vi "运维调试_总磷.vi"() -> ()   [LabVIEW 2016, in "斯坦道总磷.lvlib"]
uses:
  <vilib>/Utility/miscctls.llb/LVPointTypeDef.ctl
  <vilib>/Utility/config.llb/NI_LVConfig.lvlib
  <vilib>/ptbypt/NI_PtbyPt.lvlib
panel:
  in  "定时设置":cluster{"启动":bool, "控制命令":T1, "测量参数":T2}(xcontrol)
  in  "仪器参数设置":bool
  in  "模块启用":bool
  in  "串口设置":bool
  in  "备用系数一键写入":bool
  in  "公式一键写入":bool
  in  "流程路径":path=path "C:/Users/STD/Documents/斯坦道流程文件/流程.xml"
  in  "曲线模型":cluster{"X^2":dbl, "X":dbl, "B":dbl, "r^2":dbl}(xcontrol)
  out "字符串":string
  in  "质控参数设置":bool
  in  "总磷自动测试量程配置":T3
  out "温度2":sgl
  out "温度1":sgl
  out "ADC":sgl
  out "固件版本号":string
  in  "数组":string[](array[string])
  in  "备用系数写入":bool
  in  "备用系数读取":bool
  in  "备用系数":T4
  in  "量程切换阈值写入":bool
  in  "量程切换阈值读取":bool
  in  "量程切换阈值":cluster{"阈值":dbl, "标液浓度":dbl}
  in  "参数下拉列表":enum16{"总磷", "总氮"}(ring)
  in  "量程下拉列表":enum16{"低量程", "高量程"}(ring)
  in  "测量模式下拉列表":enum16{"水样测量", "零点核查", "跨度核查", "标样核查", "加标回收"}(ring)
  in  "公式":cluster{"X^2":dbl, "X":dbl, "b":dbl}
  in  "写公式":bool
  in  "读公式":bool
  in  "返回":bool
  in  "设置":bool
  out "序列号":string="序列号"
  out "测量数据":T5(xcontrol)
  out "集成报警信息":string
  out "总磷总氮运行状态":T6(xcontrol)
  in  "停止":bool
  in  "手动启动":bool
  in  "单步测试":bool
  in  "总磷氨氮调试":u16[](xcontrol)
  out "F3":sgl format="%#.6f"
  out "F2":sgl format="%#.6f"
  out "F1":sgl format="%#.6f"
  out "F0":sgl format="%#.6f"
  out "多列列表框":i32(listbox)
  # "参数设置"
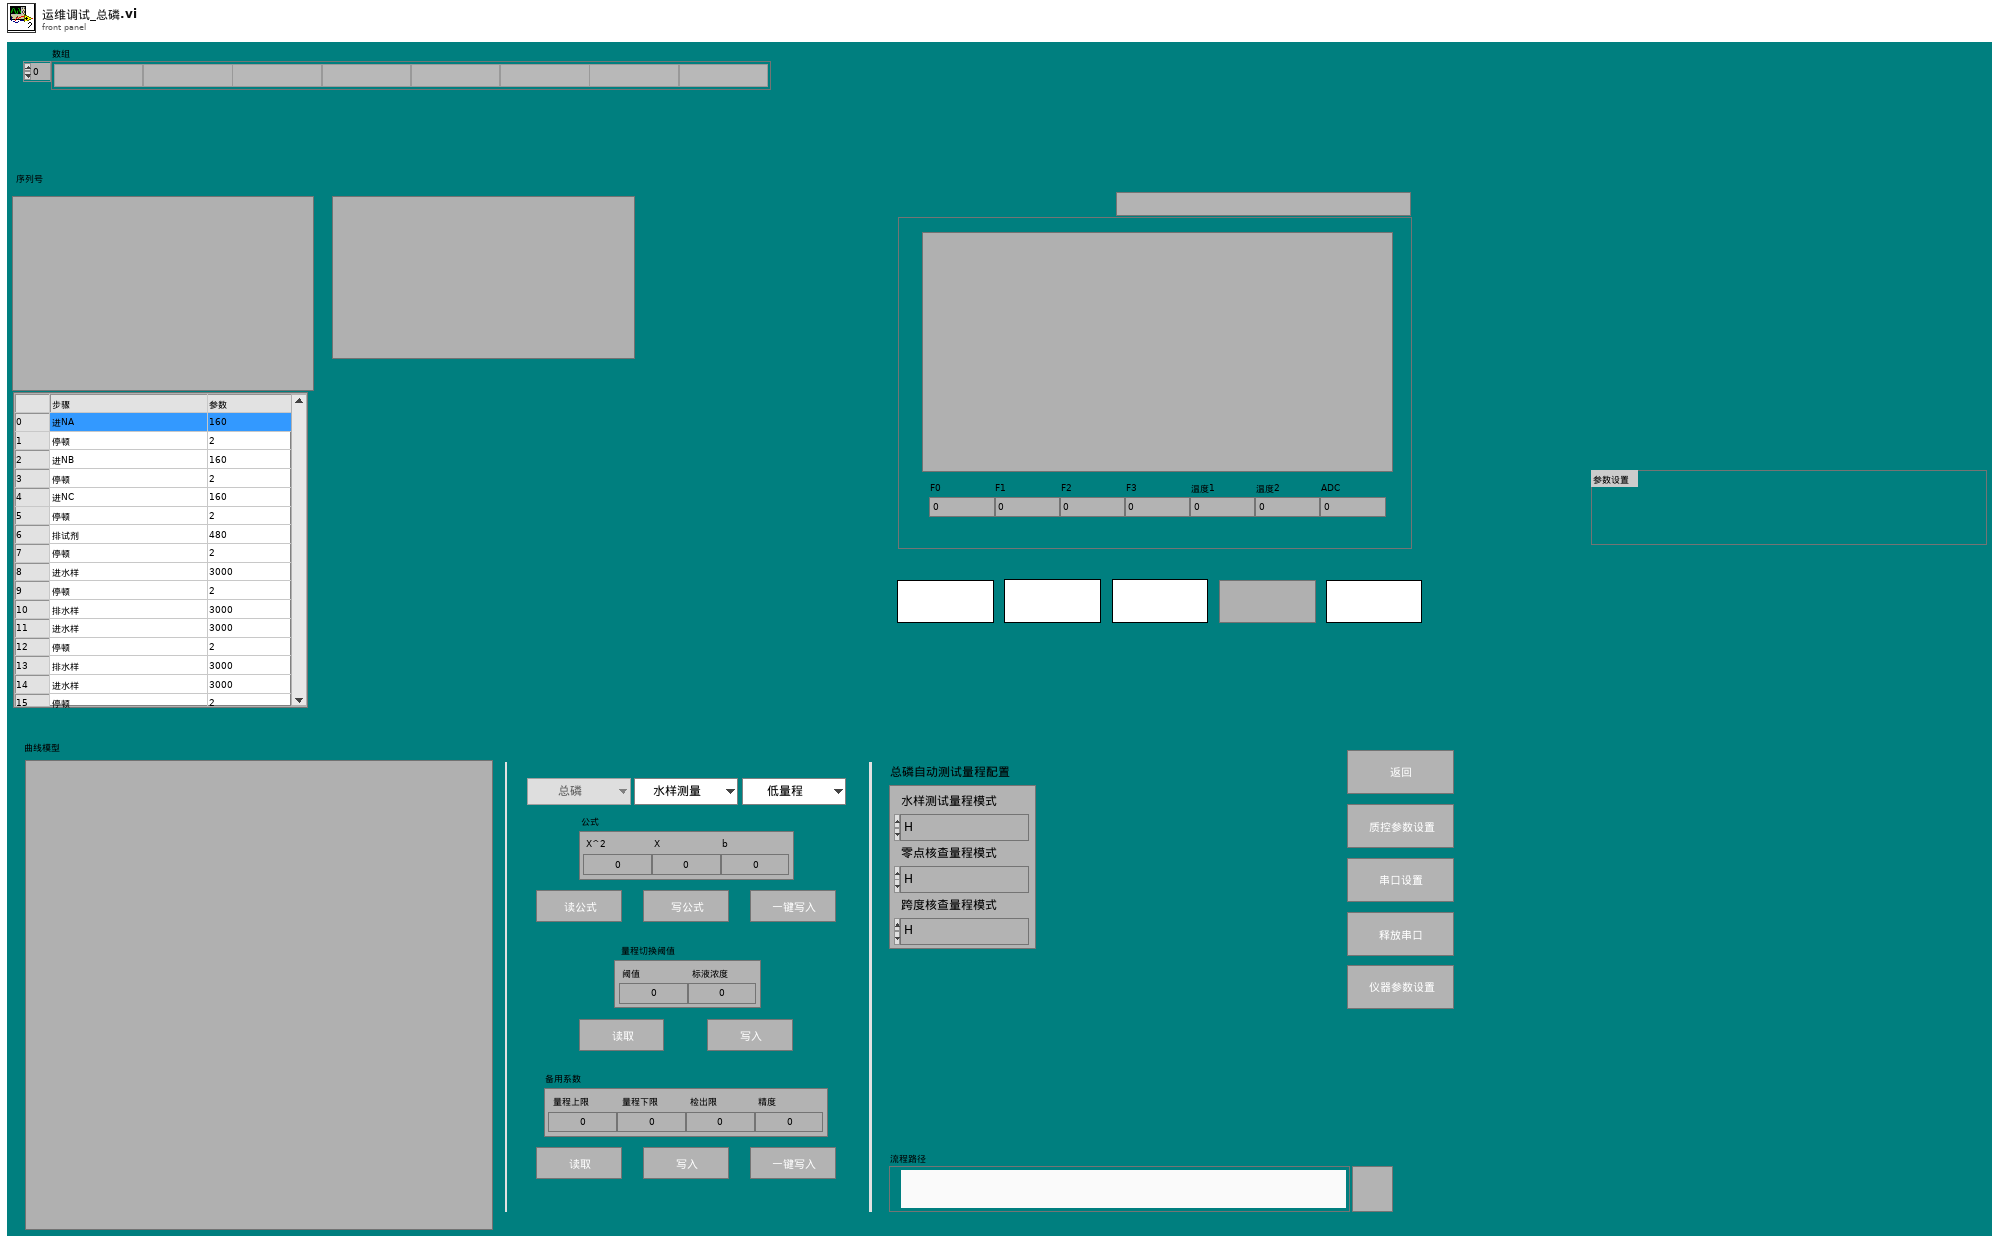
[diagram p1: front panel]
types:
  T1 = typedef "定时设置.xctl/国标控制命令.ctl" = enum16{"启动测量", "标样核查", "零点核查", "跨度核查", "空白测试", "平行样测试", "加标回收", "空白校准", "标样校准", "初始化（清洗）", "停止测试", "仪器重启", "校时", "模式设置", "测量间隔设置"}
  T2 = typedef "定时设置.xctl/测量参数.ctl" = u16
  T3 = cluster{"水样测试量程模式":enum16{"H", "L", "AUTO"}, "空白核查量程模式":enum16{"H", "L", "AUTO"}, "跨度核查量程模式":enum16{"H", "L", "AUTO"}}
  T4 = cluster{"量程上限":dbl, "量程下限":dbl, "检出限":dbl, "精度":dbl}
  T5 = cluster{"flowid":u16, "测量精度":u16, "测量数据区":cluster{"因子编码":u32, "单位":u16, "标样参考值":sgl, "水样数据时间":timestamp, "水样实测值":sgl, "水样数据标识":string, "标样数据时间":timestamp, "标样实测值":sgl, "标样数据标识":string, "空白数据时间":timestamp, "空白实测值":sgl, "空白数据标识":string, "零点核查数据时间":timestamp, "零点核查实测值":sgl, "零点核查数据标识":string, "跨度核查数据时间":timestamp, "跨度核查实测值":sgl, "跨度核查数据标识":string, "加标回收数据时间":timestamp, "加标回收实测值":sgl, "加标回收数据标识":string, "平行样数据时间":timestamp, "平行样实测值":sgl, "平行样数据标识":string, "F0":sgl, "F1":sgl, "F2":sgl, "F3":sgl, "F4":sgl, "F5":sgl, "F6":sgl, "F7":sgl, "温度":sgl, "湿度":sgl, "X值":sgl}}
  T6 = cluster{"系统时间":timestamp, "工作状态":enum16{"空闲", "水样测试", "标样核查", "零点核查", "跨度核查", "空白测试", "平行样测试", "加标回收", "空白校准", "标样校准", "初始化（清洗）"}, "测量模式":enum16{"待机", "连续模式", "周期模式", "定点模式", "受控模式", "手动模式"}, "告警代码":u16, "故障代码":u16, "日志代码":u16, "软件版本":u16, "F0":sgl, "F1":sgl, "F2":sgl, "F3":sgl, "T":sgl, "H":sgl, "id":u16, "flowid":u16, "量程":u16, "总磷控温温度1":sgl, "营养盐控温温度2":sgl, "ADC":sgl}
  T7 = typedef "NI_LVConfig.lvlib/Config Data RefNum.ctl" = refnum<k1>
  T8 = typedef "LVPointTypeDef.ctl" = cluster{"Horizontal":i16, "Vertical":i16}
  T9 = enum16{"空闲", "水样测试", "标样核查", "零点核查", "跨度核查", "空白测试", "平行样测试", "加标回收", "空白校准", "标样校准", "初始化（清洗）"}
  T10 = cluster{"因子编码":u32, "单位":u16, "标样参考值":sgl, "水样数据时间":timestamp, "水样实测值":sgl, "水样数据标识":string, "标样数据时间":timestamp, "标样实测值":sgl, "标样数据标识":string, "空白数据时间":timestamp, "空白实测值":sgl, "空白数据标识":string, "零点核查数据时间":timestamp, "零点核查实测值":sgl, "零点核查数据标识":string, "跨度核查数据时间":timestamp, "跨度核查实测值":sgl, "跨度核查数据标识":string, "加标回收数据时间":timestamp, "加标回收实测值":sgl, "加标回收数据标识":string, "平行样数据时间":timestamp, "平行样实测值":sgl, "平行样数据标识":string, "F0":sgl, "F1":sgl, "F2":sgl, "F3":sgl, "F4":sgl, "F5":sgl, "F6":sgl, "F7":sgl, "温度":sgl, "湿度":sgl, "X值":sgl}
  T11 = cluster{"时间源选择":enum16{"系统时间源", "仪器时间源"}, "外部时间源":timestamp}
  T12 = enum32{"Bad", "Idle", "Run top level", "Running"}
  T13 = cluster{"参数下拉列表":enum16{"总磷", "总氮"}, "测量模式下拉列表":enum16{"水样测量", "零点核查", "跨度核查", "标样核查", "加标回收"}, "量程下拉列表":enum16{"低量程", "高量程"}}
  T14 = cluster{"启动模式":enum16{"跨度核查", "水样测量", "空白核查", "标样核查", "加标回收"}, "启动参数":u16, "量程":enum16{"低量程", "高量程"}}
  T15 = cluster{"时间标识":timestamp, "设备":string, "日志信息":string, "流程参数":string}
  T16 = cluster{"时间标识":timestamp, "设备":string, "日志信息":string}
  T17 = typedef "LVRowAndColumnUnsignedTypeDef.ctl" = cluster{"Row":u32, "Column":u32}
  T18 = enum8{"Enabled", "Disabled", "Disabled and Grayed Out"}
  T19 = cluster{"站号":u16, "量程切换":enum32{"H", "L", "AUTO"}, "控制命令":enum16{"启动测量", "标样核查", "零点核查", "跨度核查", "空白测试", "平行样测试", "加标回收", "空白校准", "标样校准", "初始化（清洗）", "停止测试", "仪器重启", "校时", "模式设置", "测量间隔设置"}, "模式设置":enum16{"待机", "连续模式", "周期模式", "定点模式", "受控模式", "手动模式"}, "测量间隔":u16}
  T20 = cluster{"总磷跨度值":dbl, "总磷零点标准液浓度":dbl, "总磷跨度标准液浓度":dbl, "总磷标准液标准浓度":dbl}
  T21 = cluster{"确定":bool, "总磷跨度值":dbl, "总磷零点标准液浓度":dbl, "总磷跨度标准液浓度":dbl, "总磷标准液标准浓度":dbl}
  T22 = cluster{"测量量程":dbl, "测量精度":dbl, "测量间隔":dbl, "消解温度":dbl, "消解时长":dbl, "空白校准时间":timestamp, "曲线截距":dbl, "曲线斜率":dbl, "测量检出限":dbl, "测量信号值":dbl, "线性相关系数":dbl, "二次多项式系数":dbl, "标样校准时间":timestamp, "稀释倍数":dbl, "三项式系数":dbl, "空白标定系数":dbl, "量程系数":dbl, "F0/ORPA":dbl, "F1/ORPB":dbl, "F2/ORPK":dbl, "F3":dbl, "F4":dbl, "F5":dbl, "F6":dbl, "F7":dbl, "X0/滴定数":dbl, "量程":dbl}
  T23 = cluster{"确定":bool, "测量量程":dbl, "测量精度":dbl, "测量间隔":dbl, "消解温度":dbl, "消解时长":dbl, "空白校准时间":timestamp, "曲线截距":dbl, "曲线斜率":dbl, "测量检出限":dbl, "测量信号值":dbl, "线性相关系数":dbl, "二次多项式系数":dbl, "标样校准时间":timestamp, "稀释倍数":dbl, "三项式系数":dbl, "空白标定系数":dbl, "量程系数":dbl, "F0/ORPA":dbl, "F1/ORPB":dbl, "F2/ORPK":dbl, "F3":dbl, "F4":dbl, "F5":dbl, "F6":dbl, "F7":dbl, "X0/滴定数":dbl, "量程":dbl}
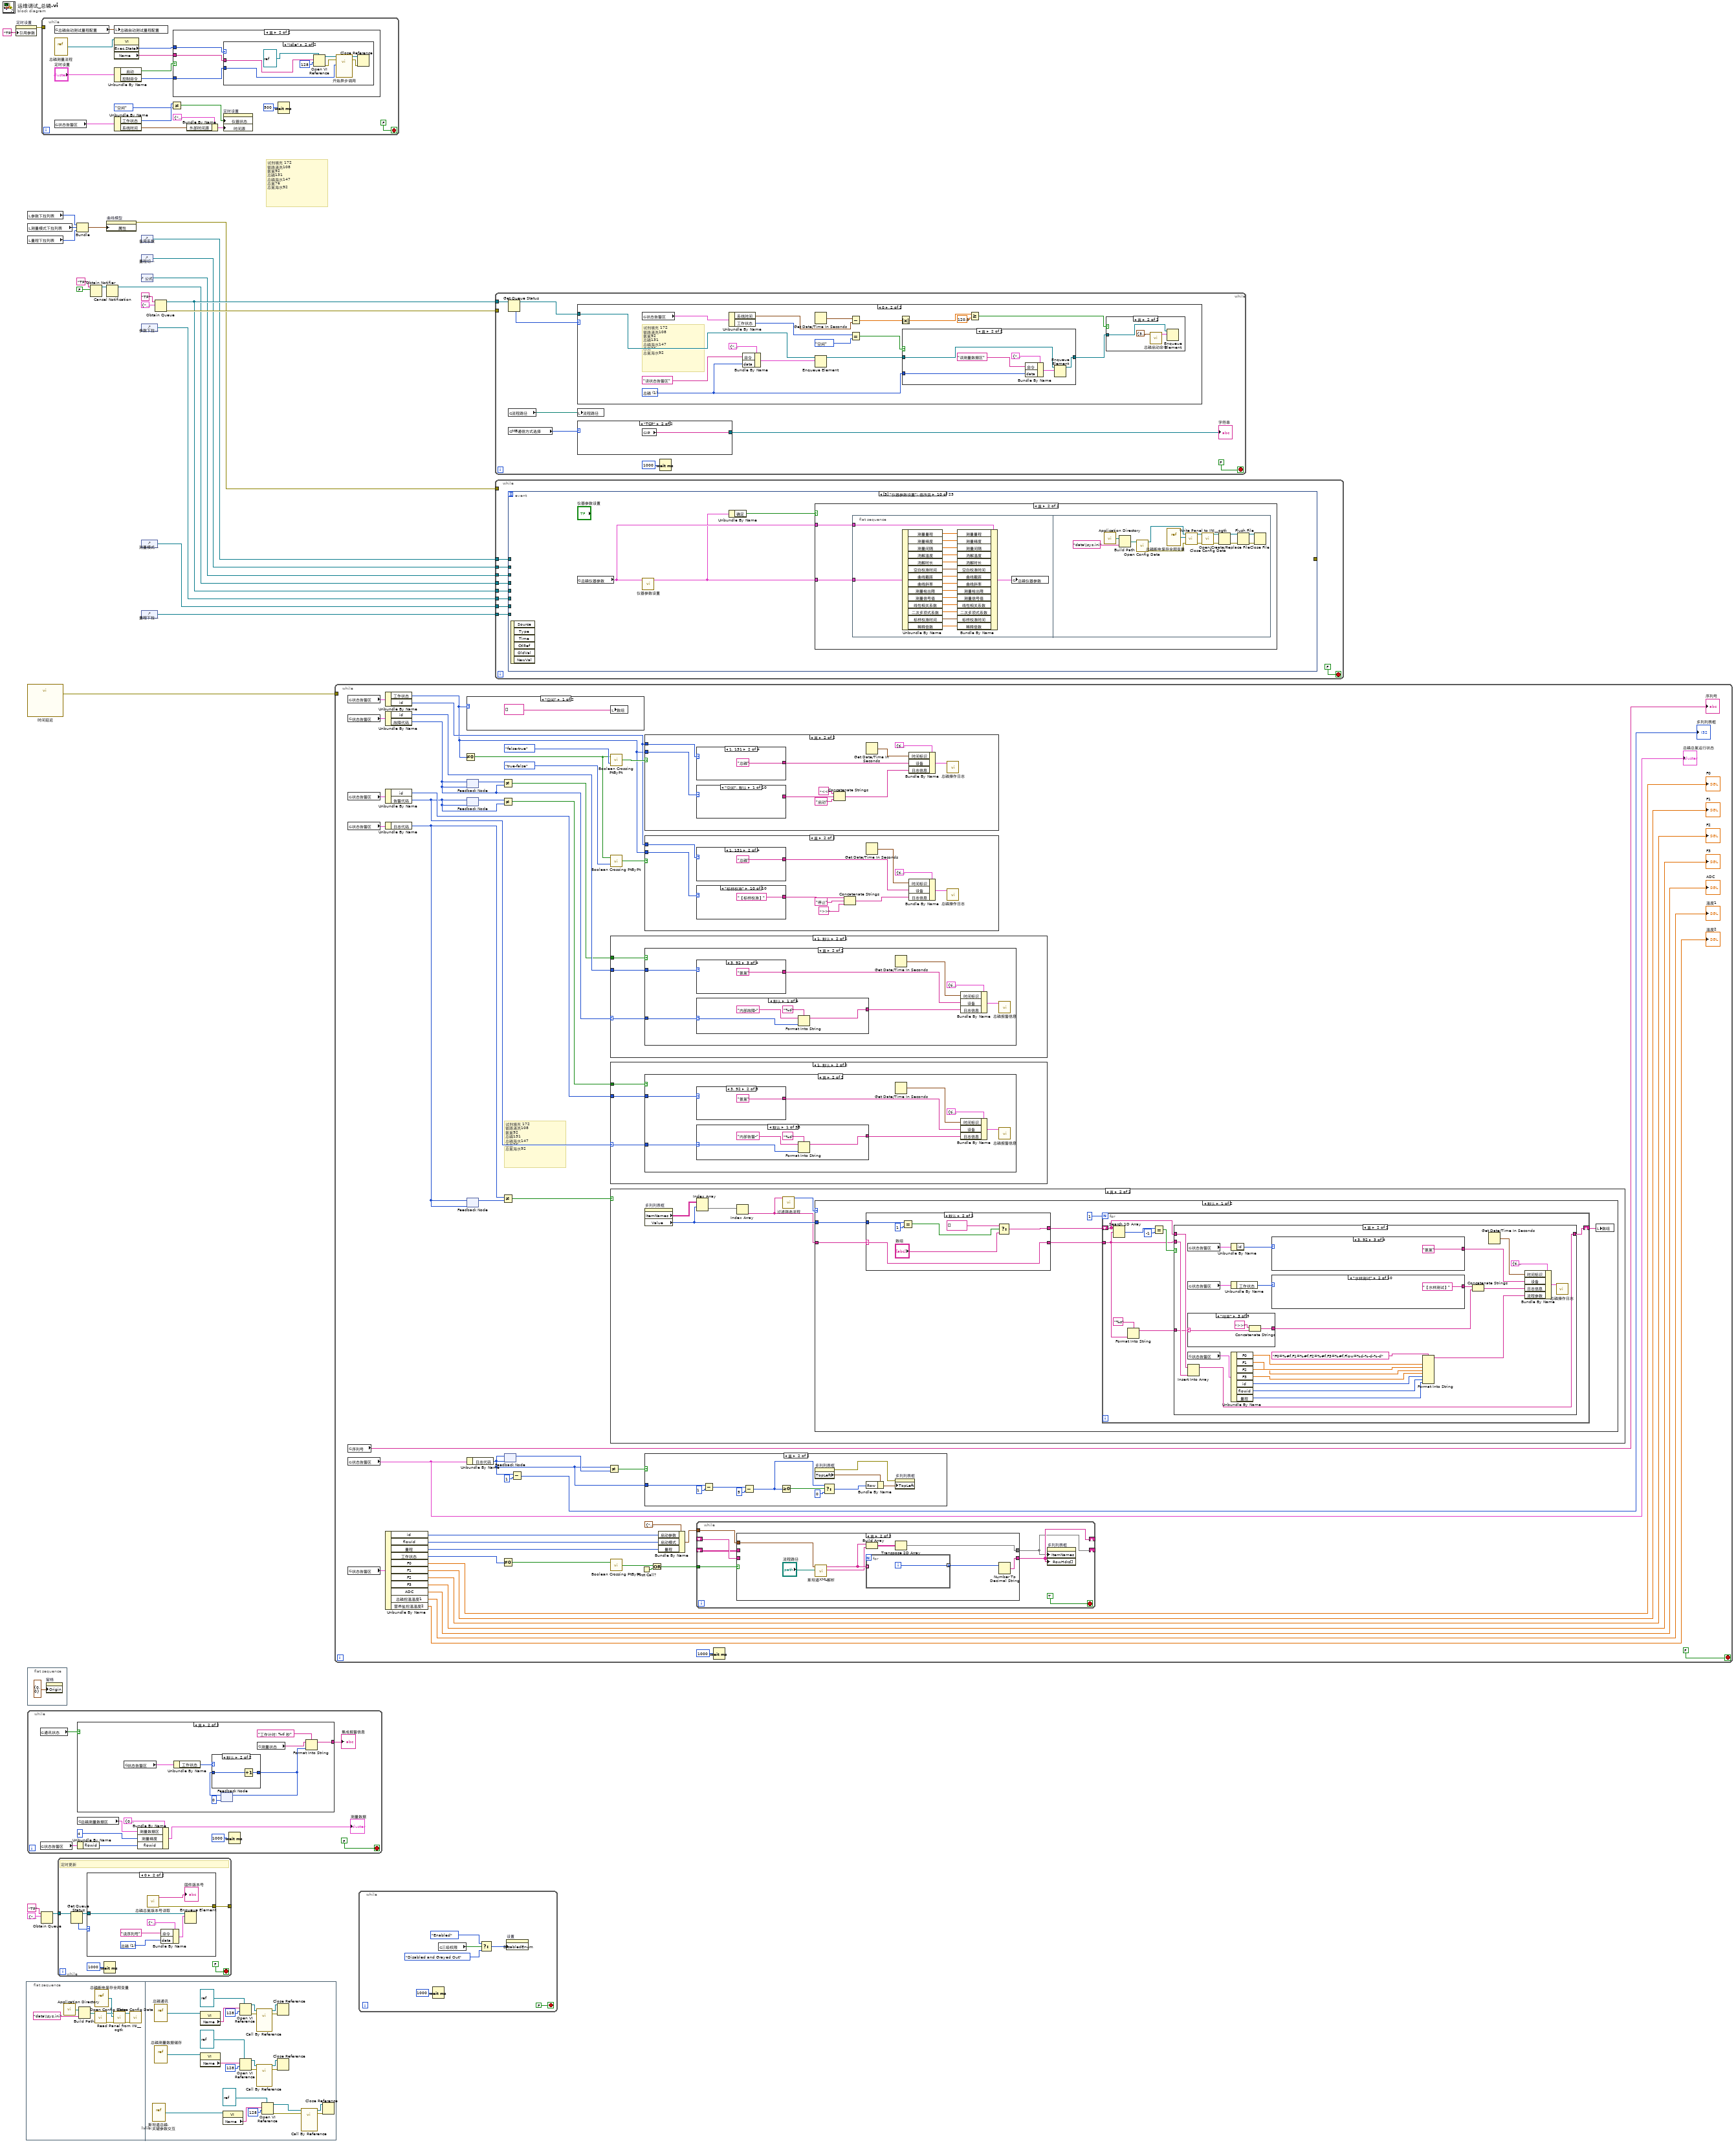
[diagram p0: block diagram]
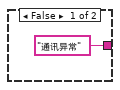
[diagram p3: hidden frame]
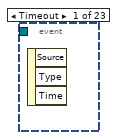
[diagram p7: hidden frame]
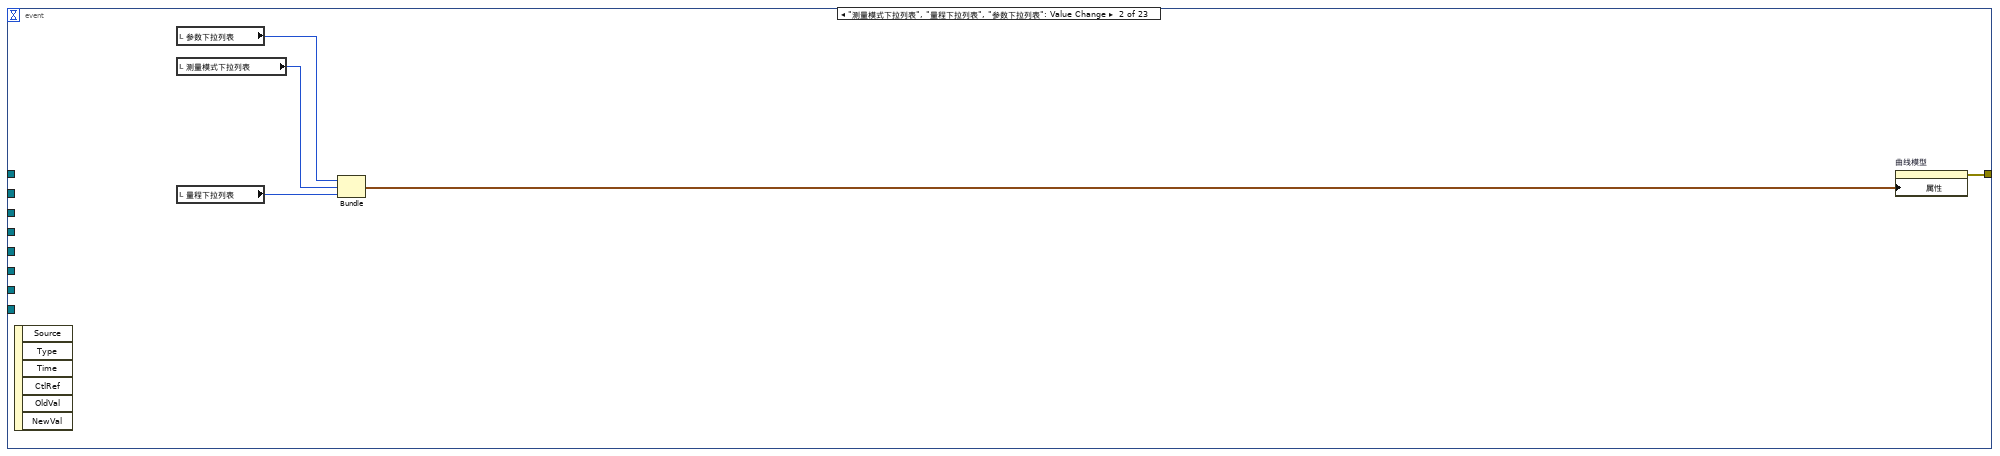
[diagram p8: hidden frame]
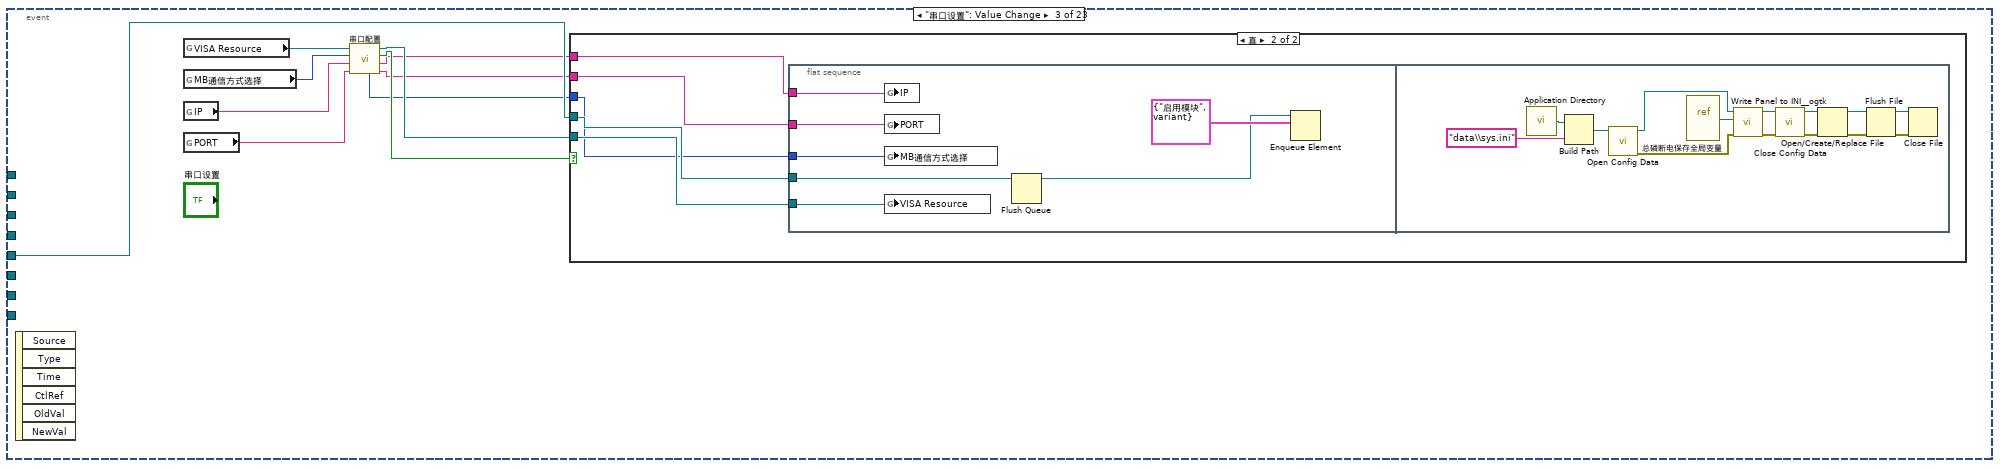
[diagram p9: hidden frame]
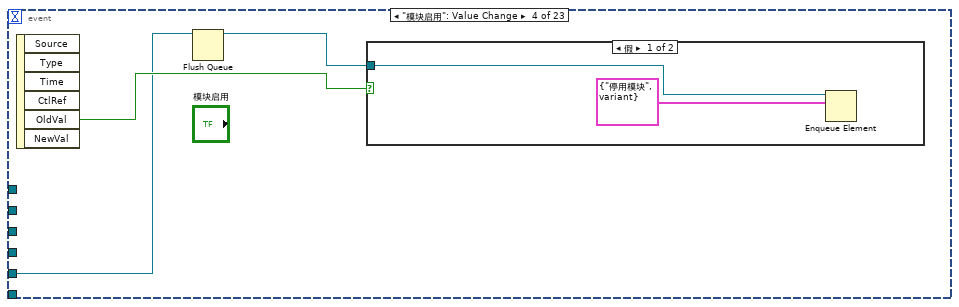
[diagram p11: hidden frame]
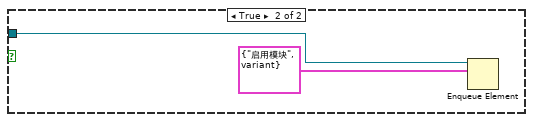
[diagram p12: hidden frame]
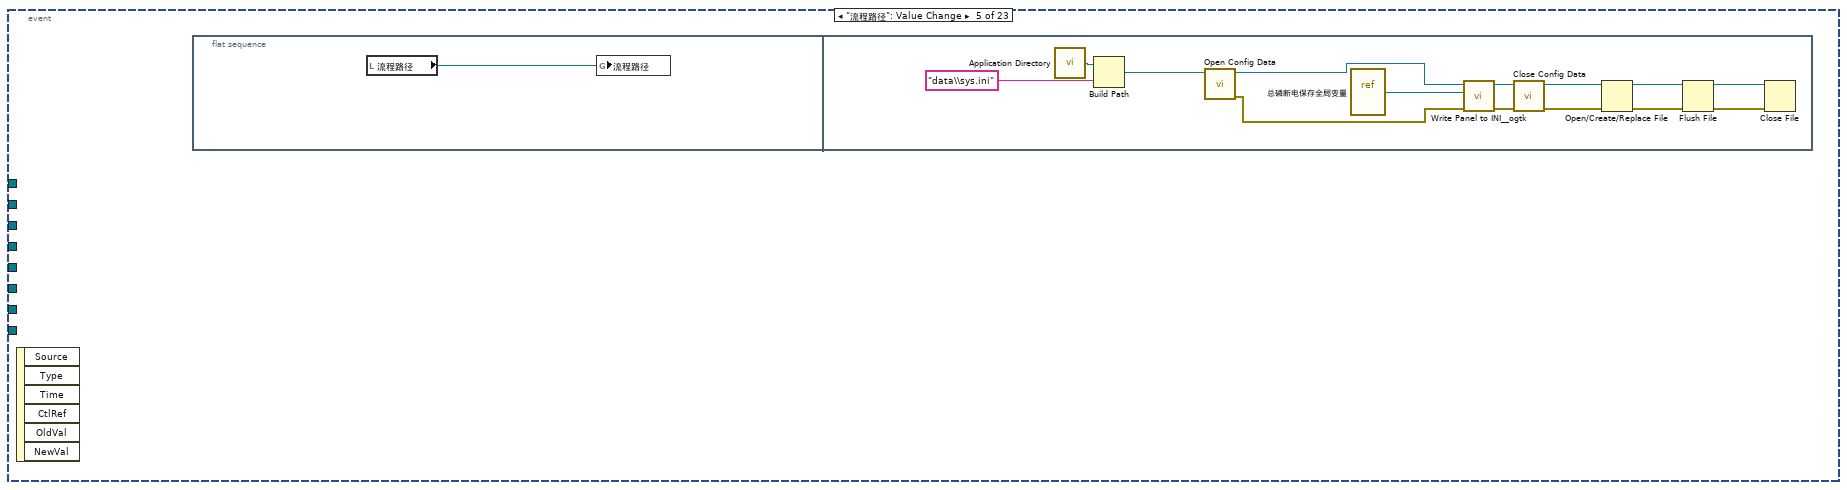
[diagram p13: hidden frame]
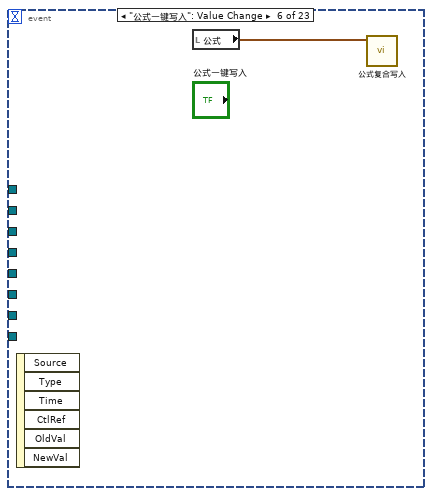
[diagram p14: hidden frame]
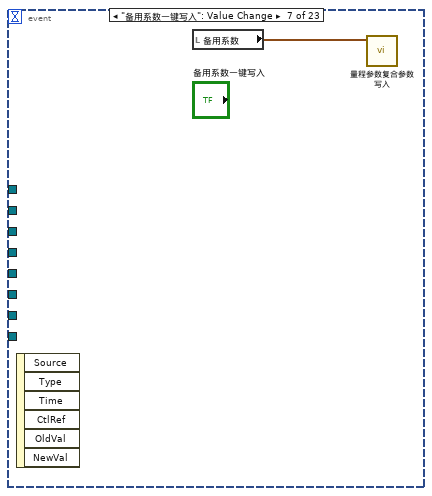
[diagram p15: hidden frame]
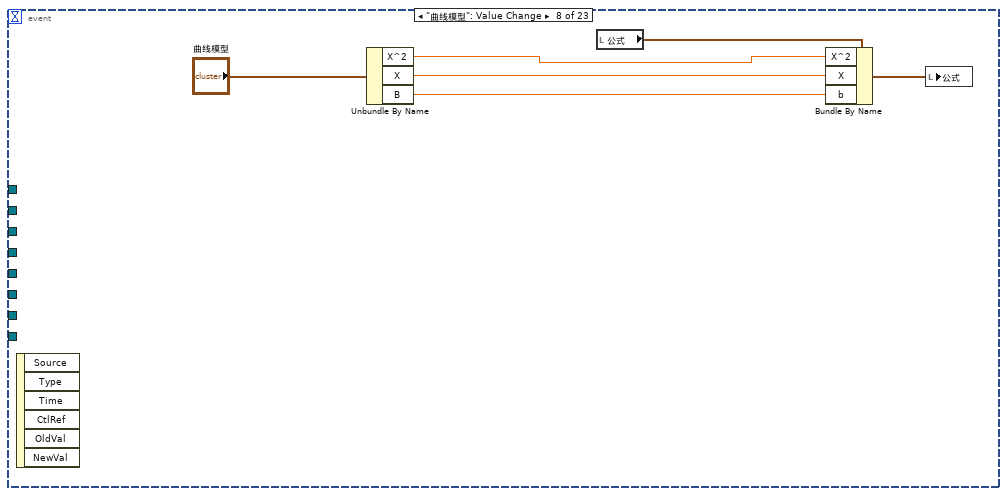
[diagram p16: hidden frame]
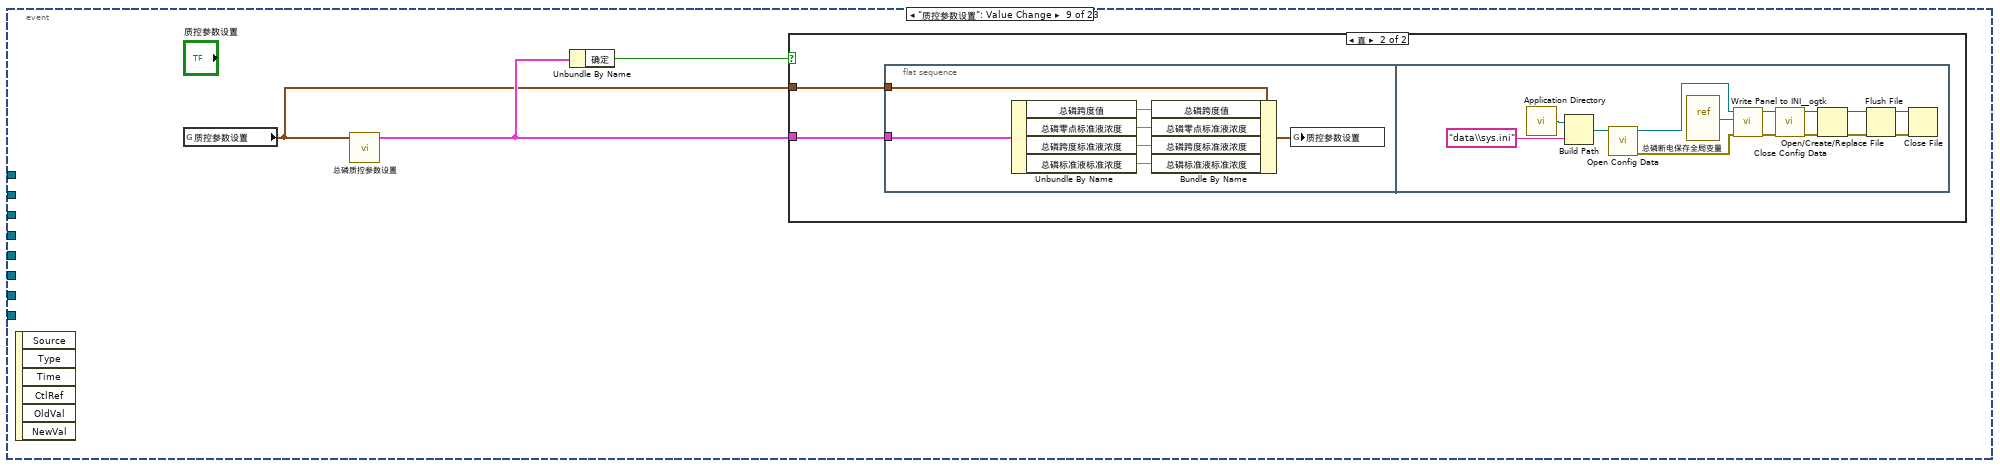
[diagram p17: hidden frame]
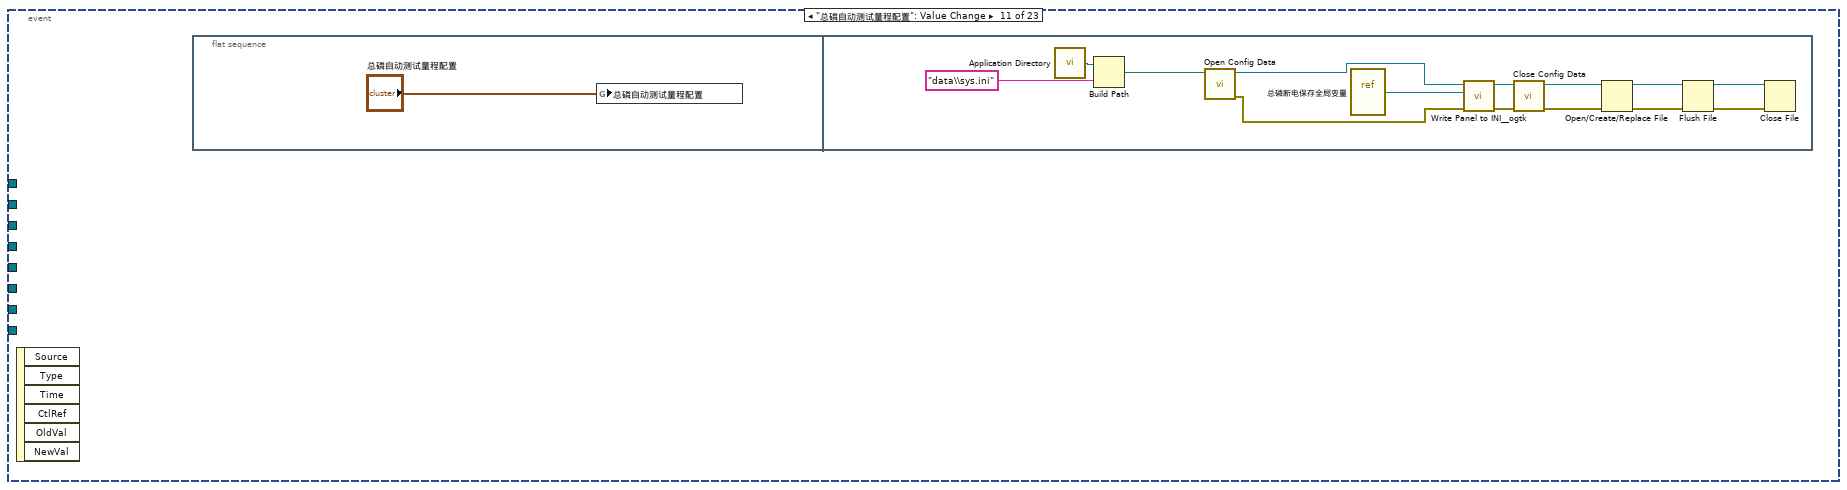
[diagram p20: hidden frame]
diagram:
  # "试剂填充 172 \n管路清洗108\n氨氮92\n总磷131\n总磷海水147\n总氮76\n总氮海水92"
  n1 = property on="定时设置" class="定时设置 (严格)"("引用参数"="TP") -> (error out=w1:errorcluster)  [unwired: 2 in, 1 out]
  n2 = flat-sequence {
    frame #0 {
      n3 = call <vilib>:"Application Directory.vi"() -> ("Application Directory"=w33:path)
      n4 = Build Path(base path=w33, name or relative path="data\\sys.ini" ("名称或相对路径")) -> (appended path=w31:path)
      n5 = vi-ref "总磷断电保存全局变量.vi"() -> (w29:refnum<vi>)
      n6 = call <vilib>:"Open Config Data.vi"("configuration file path"=w31) -> ("error out"=w27:errorcluster, "refnum"=w30:T7)  [unwired: 8 in, 1 out]
      n7 = call <userlib>:"Read Panel from INI__ogtk.vi"("error in (no error)"=w27, "VI ref"=w29, "refnum"=w30) -> ("error out"=w26:errorcluster, "refnum out"=w28:T7)  [unwired: 7 in]
      n8 = call <vilib>:"Close Config Data.vi"("error in (no error)"=w26, "refnum"=w28) -> ()  [unwired: 8 in, 2 out]
    }
    frame #1 {
      n9 = vi-ref "斯坦道总磷.lvlib:关键参数交互.vi"() -> (w34:refnum<vi>)
      n10 = vi-ref "总磷通讯.vi"() -> (w57:refnum<vi>)
      n11 = vi-ref "总磷测量数据储存.vi"() -> (w49:refnum<vi>)
      n12 = property class="VI"(reference=w57) -> ("Name"=w56:string)  [unwired: 1 in, 2 out]
      n13 = property class="VI"(reference=w49) -> ("Name"=w42:string)  [unwired: 1 in, 2 out]
      n14 = property class="VI"(reference=w34) -> ("Name"=w41:string)  [unwired: 1 in, 2 out]
      n15 = Open VI Reference(type specifier VI Refnum (for type only)=refnum<vi> refnum, vi path=w56, options=128 ("选项")) -> (vi reference=w54:refnum<vi>, error out=w52:errorcluster)  [unwired: 3 in]
      n16 = Open VI Reference(type specifier VI Refnum (for type only)=refnum<vi> refnum, vi path=w42, options=128 ("选项")) -> (vi reference=w44:refnum<vi>, error out=w46:errorcluster)  [unwired: 3 in]
      n17 = call-by-ref "?"(reference=w54, error in=w52) -> (reference out=w50:refnum<vi>, error out=w51:errorcluster)  [unwired: 12 in]
      n18 = call-by-ref "?"(reference=w44, error in=w46) -> (reference out=w48:refnum<vi>, error out=w47:errorcluster)  [unwired: 12 in]
      n19 = Open VI Reference(type specifier VI Refnum (for type only)=refnum<vi> refnum, vi path=w41, options=128 ("选项")) -> (vi reference=w39:refnum<vi>, error out=w37:errorcluster)  [unwired: 3 in]
      n20 = Close Reference(reference=w50, error in (no error)=w51) -> ()  [unwired: 1 out]
      n21 = Close Reference(reference=w48, error in (no error)=w47) -> ()  [unwired: 1 out]
      n22 = call-by-ref "?"(reference=w39, error in=w37) -> (reference out=w35:refnum<vi>, error out=w36:errorcluster)  [unwired: 12 in]
      n23 = Close Reference(reference=w35, error in (no error)=w36) -> ()  [unwired: 1 out]
    }
  }
  n24 = local read "参数下拉列表"() -> (w5:enum16{"总磷", "总氮"})
  n25 = local read "测量模式下拉列表"() -> (w4:enum16{"水样测量", "零点核查", "跨度核查", "标样核查", "加标回收"})
  n26 = local read "量程下拉列表"() -> (w3:enum16{"低量程", "高量程"})
  n27 = call "时间延迟"() -> ("error out"=w15:errorcluster)  [unwired: 11 in]
  n28 = flat-sequence {
    frame #0 {
      n29 = property on="窗格" class="Pane"("Origin"=T8 {"Horizontal"=0, "Vertical"=0} ("原点")) -> ()  [unwired: 2 in, 2 out]
    }
  }
  n30 = while {
    stop <- FALSE stop-if-true
    n31 = global read "VAR总磷全局变量.vi" "通讯状态"() -> (w66:bool)
    n32 = global read "VAR总磷全局变量.vi" "状态告警区"() -> (w64:T6)
    n33 = case shown="真" w66 {
      tunnel: ["通讯异常" ("集成报警信息") w71] -> w65
      frame False {
      }
      frame True {
        n34 = global read "VAR总磷全局变量.vi" "状态告警区"() -> (w77:T6)
        n35 = Unbundle By Name(w77) -> ("工作状态"=w76:T9)
        n36 = feedback #1(0) -> (w74:i32)
        n37 = case shown="默认" w76 {
          tunnel: w74 -> [_ w79]
          tunnel: [_ w78] -> w72
          frame "空闲" {
          }
          frame Default {
            n38 = Increment(x=w79) -> (x+1=w78:i32)
          }
        }
        n39 = feedback-in #1(w72) -> ()
        n40 = global read "VAR总磷全局变量.vi" "测量状态"() -> (w70:string)
        n41 = Format Into String(format string="工作计时: %d 秒" ("格式字符串"), initial string=w70, w72) -> (resulting string=w71:string)  [unwired: 1 in, 1 out]
      }
    }
    "集成报警信息" <- w65
    n42 = global read "VAR总磷全局变量.vi" "总磷测量数据区"() -> (w59:T10)
    n43 = Unbundle By Name(w64) -> ("flowid"=w63:u16)
    n44 = Bundle By Name(cluster=T5 {"flowid"=0, "测量精度"=0, "测量数据区"={"因子编码"=0, "单位"=0, "标样参考值"=0.0, "水样数据时间"=timestamp(0 s since 1904-01-01), "水样实测值"=0.0, "水样数据标识"="", "标样数据时间"=timestamp(0 s since 1904-01-01), "标样实测值"=0.0, "标样数据标识"="", "空白数据时间"=timestamp(0 s since 1904-01-01), "空白实测值"=0.0, "空白数据标识"="", "零点核查数据时间"=timestamp(0 s since 1904-01-01), "零点核查实测值"=0.0, "零点核查数据标识"="", "跨度核查数据时间"=timestamp(0 s since 1904-01-01), "跨度核查实测值"=0.0, "跨度核查数据标识"="", "加标回收数据时间"=timestamp(0 s since 1904-01-01), "加标回收实测值"=0.0, "加标回收数据标识"="", "平行样数据时间"=timestamp(0 s since 1904-01-01), "平行样实测值"=0.0, "平行样数据标识"="", "F0"=0.0, "F1"=0.0, "F2"=0.0, "F3"=0.0, "F4"=0.0, "F5"=0.0, "F6"=0.0, "F7"=0.0, "温度"=0.0, "湿度"=0.0, "X值"=0.0}} ("总氮测量数据"), "测量数据区"=w59, "测量精度"=u16 4, "flowid"=w63) -> (→"测量数据":T5)
    n45 = Wait (ms)(milliseconds to wait=u32 1000 ("等待时间（毫秒）")) -> ()  [unwired: 1 out]
  }
  n46 = Obtain Queue(name (unnamed)="TP" ("名称（未命名）"), element data type=cluster{"命令":string, "data":variant} {"命令"="", "data"=variant}) -> (queue out=w12:refnum<queue>)  [unwired: 3 in, 2 out]
  n47 = while {
    tunnel: w1 -> [_]
    stop <- FALSE stop-if-true
    n48 = global read "总磷断电保存全局变量.vi" "总磷自动测试量程配置"() -> (w93:T3)
    n49 = vi-ref "总磷测量流程.vi"() -> (w92:refnum<vi>)
    n50 = global read "VAR总磷全局变量.vi" "状态告警区"() -> (w86:T6)
    n51 = local write "总磷自动测试量程配置"(w93) -> ()
    n52 = property class="VI"(reference=w92) -> ("Exec.State"=w91:T12, "Name"=w90:string)  [unwired: 1 in, 2 out]
    n53 = Unbundle By Name("定时设置") -> ("启动"=w88:bool, "控制命令"=w87:T1)
    n54 = Unbundle By Name(w86) -> ("工作状态"=w85:T9, "系统时间"=w80:timestamp)
    n55 = Not Equal?(x=w85, y=T9."空闲") -> (x != y?=w83:bool)
    n56 = case shown="真" w88 {
      tunnel: w90 -> [_ w98]
      tunnel: w91 -> [_ w97]
      tunnel: w87 -> [_ w96]
      frame False {
      }
      frame True {
        n57 = case shown="\"Idle\"" w97 {
          tunnel: w98 -> [_ w102]
          tunnel: w96 -> [_ w99]
          frame "Bad", Default {
          }
          frame "Idle" {
            n58 = Open VI Reference(type specifier VI Refnum (for type only)=refnum<vi> refnum, vi path=w102, options=128 ("选项")) -> (vi reference=w103:refnum<vi>, error out=w104:errorcluster)  [unwired: 3 in]
            n59 = call-by-ref "开始异步调用"(reference=w103, error in=w104, "控制命令"=w99) -> (reference out=w105:refnum<vi>, error out=w106:errorcluster)  [unwired: 11 in]
            n60 = Close Reference(reference=w105, error in (no error)=w106) -> ()  [unwired: 1 out]
          }
        }
      }
    }
    n61 = Bundle By Name(cluster=T11 {"时间源选择"=enum."仪器时间源", "外部时间源"=timestamp(0 s since 1904-01-01)} ("时间源"), "外部时间源"=w80) -> (w81:T11)
    n62 = property on="定时设置" class="定时设置 (严格)"("仪器状态"=w83, "时间源"=w81) -> ()  [unwired: 2 in, 2 out]
    n63 = Wait (ms)(milliseconds to wait=u32 500 ("等待时间（毫秒）")) -> ()  [unwired: 1 out]
  }
  n64 = while {
    tunnel: w12 -> [w111]
    tunnel: [w109] -> _
    stop <- FALSE stop-if-true
    # "定时更新"
    n65 = Get Queue Status(queue=w111) -> (queue out=w108:refnum<queue>, # elements in queue=w107:i32)  [unwired: 2 in, 6 out]
    n66 = case shown="0" w107 {
      tunnel: w108 -> [_ w116]
      tunnel: [_ w113] -> w109
      frame Default {
      }
      frame 0 {
        w117 = u16 1 items=["总磷"=1, "氨氮"=3] ("站号")
        n67 = call "总磷总氮版本号读取.vi"() -> ("error out"=w113:errorcluster, "固件版本号"=→"固件版本号":string)  [unwired: 10 in]
        n68 = Bundle By Name(cluster=cluster{"命令":string, "data":variant} {"命令"="", "data"=variant} ("元素"), "命令"="读序列号", "data"=w117) -> (w115:cluster{"命令":string, "data":variant})
        n69 = Enqueue Element(queue=w116, element=w115) -> ()  [unwired: 2 in, 3 out]
      }
    }
    n70 = Wait (ms)(milliseconds to wait=u32 1000 ("等待时间（毫秒）")) -> ()  [unwired: 1 out]
  }
  n71 = Bundle("参数下拉列表"=w5, "测量模式下拉列表"=w4, "量程下拉列表"=w3) -> (w6:T13)  [unwired: 1 in]
  n72 = Obtain Notifier(name (unnamed)="TP" ("名称（未命名）"), notification data type=FALSE) -> (notifier out=w8:refnum<notifier>)  [unwired: 2 in, 2 out]
  n73 = property on="曲线模型" class="曲线模型 (严格)"("属性"=w6) -> (error out=w11:errorcluster)  [unwired: 2 in, 1 out]
  n74 = Cancel Notification(0:w8) -> (8:w7:refnum<notifier>)  [unwired: 1 in, 2 out]
  n75 = control-ref of="备用系数"() -> (w16:refnum<vi>)
  n76 = control-ref of="量程切换阈值"() -> (w17:refnum<vi>)
  n77 = control-ref of="公式"() -> (w18:refnum<vi>)
  n78 = control-ref of="参数下拉列表"() -> (w20:refnum<vi>)
  n79 = control-ref of="测量模式下拉列表"() -> (w19:refnum<vi>)
  n80 = control-ref of="量程下拉列表"() -> (w21:refnum<vi>)
  n81 = Obtain Queue(name (unnamed)="TP" ("名称（未命名）"), element data type=cluster{"命令":string, "data":variant} {"命令"="", "data"=variant}) -> (queue out=w22:refnum<queue>, error out=w23:errorcluster)  [unwired: 3 in, 1 out]
  n82 = while {
    tunnel: w15 -> [_]
    stop <- FALSE stop-if-true
    # "试剂填充 172 \n管路清洗108\n氨氮92\n总磷131\n总磷海水147\n总氮76\n总氮海水92"
    n83 = global read "VAR总磷全局变量.vi" "状态告警区"() -> (w140:T6)
    n84 = global read "VAR总磷全局变量.vi" "状态告警区"() -> (w145:T6)
    n85 = global read "VAR总磷全局变量.vi" "状态告警区"() -> (w150:T6)
    n86 = global read "VAR总磷全局变量.vi" "状态告警区"() -> (w138:T6)
    n87 = global read "VAR总磷全局变量.vi" "序列号"() -> (→"序列号":string)
    n88 = global read "VAR总磷全局变量.vi" "状态告警区"() -> (w153:T6)
    "总磷总氮运行状态" <- w153
    n89 = global read "VAR总磷全局变量.vi" "状态告警区"() -> (w161:T6)
    n90 = Unbundle By Name(w140) -> ("工作状态"=w120:T9, "id"=w121:u16)
    n91 = Unbundle By Name(w145) -> ("id"=w144:u16, "故障代码"=w141:u16)
    n92 = Unbundle By Name(w150) -> ("id"=w149:u16, "告警代码"=w146:u16)
    n93 = Unbundle By Name(w138) -> ("日志代码"=w137:u16)
    n94 = Unbundle By Name(w161) -> ("id"=w158:u16, "flowid"=w160:u16, "量程"=w159:u16, "工作状态"=w128:T9, "F0"=→"F0":sgl, "F1"=→"F1":sgl, "F2"=→"F2":sgl, "F3"=→"F3":sgl, "ADC"=→"ADC":sgl, "总磷控温温度1"=→"温度1":sgl, "营养盐控温温度2"=→"温度2":sgl)
    n95 = Not Equal To 0?(x=w120) -> (x != 0?=w123:bool)
    n96 = case shown="\"空闲\"" w120 {
      frame "空闲" {
        n97 = local write "数组"(string[] [] ("数组")) -> ()
      }
      frame "水样测试", Default {
      }
    }
    n98 = feedback #2(w141) -> (w142:u16)
    n99 = feedback-in #2(w141) -> ()
    n100 = feedback #3(w146) -> (w147:u16)
    n101 = feedback-in #3(w146) -> ()
    n102 = feedback #4(w137) -> (w139:u16)
    n103 = feedback-in #4(w137) -> ()
    n104 = Unbundle By Name(w153) -> ("日志代码"=w134:u16)
    n105 = Not Equal?(x=w142, y=w141) -> (x != y?=w143:bool)
    n106 = Not Equal?(x=w147, y=w146) -> (x != y?=w148:bool)
    n107 = Not Equal?(x=w137, y=w139) -> (x != y?=w136:bool)
    n108 = Not Equal To 0?(x=w128) -> (x != 0?=w163:bool)
    n109 = feedback-in #5(w134) -> ()
    n110 = feedback #5(w134) -> (w166:u16)
    n111 = Subtract(x=w134, y=1) -> (x-y=→"多列列表框":i32)
    n112 = Not Equal?(x=w134, y=w166) -> (x != y?=w165:bool)
    n113 = call <vilib>:"Boolean Crossing PtByPt.vi"("direction"=enum16{"either", "false-true", "true-false"}."false-true", "input"=w123) -> ("crossing"=w125:bool)  [unwired: 1 in]
    n114 = call <vilib>:"Boolean Crossing PtByPt.vi"("direction"=enum16{"either", "false-true", "true-false"}."true-false", "input"=w123) -> ("crossing"=w122:bool)  [unwired: 1 in]
    n115 = case shown="1, 默认" w141 {
      selector: w141 -> [_ w288]
      tunnel: w144 -> [_ w289]
      tunnel: w143 -> [_ w287]
      frame 0 {
      }
      frame 1, Default {
        n116 = case shown="真" w287 {
          tunnel: w289 -> [_ w296]
          tunnel: w288 -> [_ w291]
          frame False {
          }
          frame True {
            n117 = case shown="3, 92" w296 {
              tunnel: [_ "总磷" ("table输入") "氨氮" ("table输入") "总氮" ("table输入")] -> w292
              frame Default {
              }
              frame 1, 131 {
              }
              frame 3, 92 {
              }
              frame 2, 76 {
              }
            }
            n118 = case shown="默认" w291 {
              selector: w291 -> [w298 _ _ _ _ _]
              tunnel: [w297 "无故障" "电机故障" "温度故障" "通讯故障" "滴定故障"] -> w290
              frame Default {
                n119 = Format Into String(format string="%d" ("格式字符串"), initial string="内部故障-" ("工作状态"), w298) -> (resulting string=w297:string)  [unwired: 1 in, 1 out]
              }
              frame 0 {
              }
              frame 1 {
              }
              frame 2 {
              }
              frame 3 {
              }
              frame 4 {
              }
            }
            n120 = Get Date/Time In Seconds() -> (seconds since 1Jan1904=w293:timestamp)
            n121 = Bundle By Name(cluster=T16 {"时间标识"=timestamp(0 s since 1904-01-01), "设备"="", "日志信息"=""} ("data in"), "时间标识"=w293, "设备"=w292, "日志信息"=w290) -> (w294:T16)
            n122 = call "总磷报警信息.vi"("data in"=w294) -> ()  [unwired: 10 in, 1 out]
          }
        }
      }
    }
    n123 = case shown="1, 默认" w146 {
      selector: w146 -> [_ w310]
      tunnel: w149 -> [_ w311]
      tunnel: w148 -> [_ w309]
      frame 0 {
      }
      frame 1, Default {
        n124 = case shown="真" w309 {
          tunnel: w311 -> [_ w318]
          tunnel: w310 -> [_ w312]
          frame False {
          }
          frame True {
            n125 = case shown="3, 92" w318 {
              tunnel: ["总磷" ("table输入") "氨氮" ("table输入") "总氮" ("table输入")] -> w314
              frame 1, 131 {
              }
              frame 3, 92 {
              }
              frame 2, 76, Default {
              }
            }
            n126 = case shown="默认" w312 {
              selector: w312 -> [w320 _ _ _ _ _ _ _ _ _ _ _ _ _ _ _ _ _ _ _ _ _ _ _ _ _ _ _ _ _ _ _ _ _ _ _ _ _]
              tunnel: [w319 "无告警" "缺试剂告警" "缺水样告警" "缺蒸馏水告警" "缺标液告警" "仪表漏液告警" "标定异常告警" "超量程告警" "加热异常" "低试剂预警" "超上限告警" "超下限告警" "仪表内部其他异常" "滴定异常告警" "电极异常告警" "量程切换告警" "参数设置告警" "PH电极电位异常" "电导率电极异常" "浊度光度异常" "溶解氧电极异常" "溶解氧光强异常" "温度异常告警" "PH异常告警" "溶解氧异常告警" "电导率异常告警" "浊度异常告警" "叶绿素异常告警" "藻密度异常告警" "蓝绿藻异常告警" "ORP异常告警" "氨氮异常告警" "清洁刷异常告警" "SD卡异常告警" "蓝牙异常告警" "WiFi异常告警" "流程异常告警"] -> w313
              frame Default {
                n127 = Format Into String(format string="%d" ("格式字符串"), initial string="内部告警-" ("工作状态"), w320) -> (resulting string=w319:string)  [unwired: 1 in, 1 out]
              }
              frame 0 {
              }
              frame 1 {
              }
              frame 2 {
              }
              frame 3 {
              }
              frame 4 {
              }
              frame 5 {
              }
              frame 6 {
              }
              frame 7 {
              }
              frame 8 {
              }
              frame 9 {
              }
              frame 10 {
              }
              frame 11 {
              }
              frame 12 {
              }
              frame 13 {
              }
              frame 14 {
              }
              frame 15 {
              }
              frame 16 {
              }
              frame 17 {
              }
              frame 18 {
              }
              frame 19 {
              }
              frame 20 {
              }
              frame 21 {
              }
              frame 22 {
              }
              frame 23 {
              }
              frame 24 {
              }
              frame 25 {
              }
              frame 26 {
              }
              frame 27 {
              }
              frame 28 {
              }
              frame 29 {
              }
              frame 30 {
              }
              frame 31 {
              }
              frame 32 {
              }
              frame 33 {
              }
              frame 34 {
              }
              frame 35 {
              }
              frame 36 {
              }
            }
            n128 = Get Date/Time In Seconds() -> (seconds since 1Jan1904=w315:timestamp)
            n129 = Bundle By Name(cluster=T16 {"时间标识"=timestamp(0 s since 1904-01-01), "设备"="", "日志信息"=""} ("data in"), "时间标识"=w315, "设备"=w314, "日志信息"=w313) -> (w316:T16)
            n130 = call "总磷报警信息.vi"("data in"=w316) -> ()  [unwired: 10 in, 1 out]
          }
        }
      }
    }
    n131 = case shown="真" w136 {
      frame False {
      }
      frame True {
        n132 = property on="多列列表框" class="MCListbox (严格)"() -> ("ItemNames"=w218:string[][], "Value"=w216:i32)  [unwired: 2 in, 2 out]
        n133 = Index Array(array=w218, index (row)=w216) -> (element=w217:string[])  [unwired: 1 in]
        n134 = Index Array(array=w217) -> (element=w214:string)  [unwired: 1 in]
        n135 = call "过滤筛选流程.vi"("字符串"=w214) -> ("匹配后偏移量"=w215:i32)  [unwired: 10 in]
        n136 = case shown="默认" w215 {
          tunnel: w216 -> [w220 _]
          tunnel: w214 -> [w219 _]
          frame Default {
            n137 = case shown="默认" w219 {
              selector: w219 -> [w226 w233]
              tunnel: [w226 w233] -> w222
              tunnel: [string[] [] ("数组") w228] -> w221
              tunnel: w220 -> [_ w232]
              frame "读数" {
              }
              frame Default {
                n138 = Equal?(x=w232, y=1) -> (x = y?=w230:bool)
                n139 = Select(t=string[] [], s=w230, f="数组") -> (s? t:f=w228:string[])
              }
            }
            n140 = for {
              N: 1 -> [_]
              tunnel: w222 -> [w235]
              shift-right: [w234] -> w223
              shift-left: w221 -> [w236]
              n141 = Search 1D Array(1D array=w236, element=w235) -> (index of element=w239:i32)  [unwired: 1 in]
              n142 = Format Into String(format string="%s" ("格式字符串"), w235) -> (resulting string=w240:string)  [unwired: 2 in, 1 out]
              n143 = Equal?(x=w239, y=-1) -> (x = y?=w237:bool)
              n144 = case shown="真" w237 {
                tunnel: w240 -> [_ w248]
                tunnel: w236 -> [w242 w252]
                tunnel: w235 -> [_ w251]
                tunnel: [w242 w250] -> w234
                frame False {
                }
                frame True {
                  n145 = global read "VAR总磷全局变量.vi" "状态告警区"() -> (w267:T6)
                  n146 = global read "VAR总磷全局变量.vi" "状态告警区"() -> (w246:T6)
                  n147 = case shown="\"结束\"" w248 {
                    selector: w248 -> [w277 w280 w283]
                    tunnel: [w277 w279 w282] -> w247
                    frame Default {
                    }
                    frame "初始化" {
                      n148 = Concatenate Strings("<<" ("字符串"), w280) -> (w279:string)
                    }
                    frame "结束" {
                      n149 = Concatenate Strings(">>" ("字符串"), w283) -> (w282:string)
                    }
                  }
                  n150 = global read "VAR总磷全局变量.vi" "状态告警区"() -> (w262:T6)
                  n151 = Insert Into Array(array=w252, new element=w251) -> (w250:string[])  [unwired: 1 in]
                  n152 = Unbundle By Name(w267) -> ("id"=w266:u16)
                  n153 = Unbundle By Name(w246) -> ("工作状态"=w245:T9)
                  n154 = Unbundle By Name(w262) -> ("F0"=w259:sgl, "F1"=w258:sgl, "F2"=w257:sgl, "F3"=w256:sgl, "id"=w255:u16, "flowid"=w254:u16, "量程"=w253:u16)
                  n155 = case shown="3, 92" w266 {
                    tunnel: [_ "总磷" ("table输入") "氨氮" ("table输入") "总氮" ("table输入")] -> w264
                    frame Default {
                    }
                    frame 1, 131 {
                    }
                    frame 3, 92 {
                    }
                    frame 2, 76 {
                    }
                  }
                  n156 = case shown="\"水样测试\"" w245 {
                    tunnel: [_ "【水样测试】" ("字符串") "【标样核查】" ("字符串") "【零点核查】" ("字符串") "【跨度核查】" ("字符串") "【空白测试】" ("字符串") "【平行样测试】" ("字符串") "【加标回收】" ("字符串") "【空白校准】" ("字符串") "【标样校准】" ("字符串")] -> w243
                    frame "空闲", Default {
                    }
                    frame "水样测试" {
                    }
                    frame "标样核查" {
                    }
                    frame "零点核查" {
                    }
                    frame "跨度核查" {
                    }
                    frame "空白测试" {
                    }
                    frame "平行样测试" {
                    }
                    frame "加标回收" {
                    }
                    frame "空白校准" {
                    }
                    frame "标样校准" {
                    }
                  }
                  n157 = Format Into String(format string="F0=%#f,F1=%#f,F2=%#f,F3=%#f,Flow=%d-%-d-%-d" ("格式字符串"), w259, w258, w257, w256, w255, w254, w253) -> (resulting string=w260:string)  [unwired: 2 in, 1 out]
                  n158 = Concatenate Strings(w243, w247) -> (w244:string)
                  n159 = Get Date/Time In Seconds() -> (seconds since 1Jan1904=w263:timestamp)
                  n160 = Bundle By Name(cluster=T15 {"时间标识"=timestamp(0 s since 1904-01-01), "设备"="", "日志信息"="", "流程参数"=""} ("data in"), "时间标识"=w263, "设备"=w264, "日志信息"=w244, "流程参数"=w260) -> (w265:T15)
                  n161 = call "总磷操作日志.vi"("data in"=w265) -> ()  [unwired: 11 in]
                }
              }
            }
            n162 = local write "数组"(w223) -> ()
          }
          frame -1 {
          }
        }
      }
    }
    n163 = call <vilib>:"Boolean Crossing PtByPt.vi"("input"=w163) -> ("crossing"=w127:bool)  [unwired: 2 in]
    n164 = First Call?() -> (First Call?: T/F=w164:bool)
    n165 = case shown="真" w125 {
      tunnel: w120 -> [_ w193]
      tunnel: w121 -> [_ w192]
      frame False {
      }
      frame True {
        n166 = case shown="1, 131" w192 {
          tunnel: [_ "总磷" ("table输入") "氨氮" ("table输入") "总氮" ("table输入")] -> w198
          frame Default {
          }
          frame 1, 131 {
          }
          frame 3, 92 {
          }
          frame 2, 76 {
          }
        }
        n167 = case shown="\"空闲\", 默认" w193 {
          tunnel: [_ "【水样测试】" ("字符串") "【标样核查】" ("字符串") "【零点核查】" ("字符串") "【跨度核查】" ("字符串") "【空白测试】" ("字符串") "【平行样测试】" ("字符串") "【加标回收】" ("字符串") "【空白校准】" ("字符串") "【标样校准】" ("字符串")] -> w197
          frame "空闲", Default {
          }
          frame "水样测试" {
          }
          frame "标样核查" {
          }
          frame "零点核查" {
          }
          frame "跨度核查" {
          }
          frame "空白测试" {
          }
          frame "平行样测试" {
          }
          frame "加标回收" {
          }
          frame "空白校准" {
          }
          frame "标样校准" {
          }
        }
        n168 = Concatenate Strings("<<" ("字符串"), w197, "启动" ("字符串")) -> (w194:string)
        n169 = Get Date/Time In Seconds() -> (seconds since 1Jan1904=w200:timestamp)
        n170 = Bundle By Name(cluster=T15 {"时间标识"=timestamp(0 s since 1904-01-01), "设备"="", "日志信息"="", "流程参数"=""} ("data in"), "时间标识"=w200, "设备"=w198, "日志信息"=w194) -> (w191:T15)
        n171 = call "总磷操作日志.vi"("data in"=w191) -> ()  [unwired: 11 in]
      }
    }
    n172 = case shown="真" w122 {
      tunnel: w120 -> [_ w172]
      tunnel: w121 -> [_ w171]
      frame False {
      }
      frame True {
        n173 = case shown="1, 131" w171 {
          tunnel: [_ "总磷" ("table输入") "氨氮" ("table输入") "总氮" ("table输入")] -> w176
          frame Default {
          }
          frame 1, 131 {
          }
          frame 3, 92 {
          }
          frame 2, 76 {
          }
        }
        n174 = case shown="\"标样校准\"" w172 {
          tunnel: [_ "【水样测试】" ("字符串") "【标样核查】" ("字符串") "【零点核查】" ("字符串") "【跨度核查】" ("字符串") "【空白测试】" ("字符串") "【平行样测试】" ("字符串") "【加标回收】" ("字符串") "【空白校准】" ("字符串") "【标样校准】" ("字符串")] -> w175
          frame "空闲", Default {
          }
          frame "水样测试" {
          }
          frame "标样核查" {
          }
          frame "零点核查" {
          }
          frame "跨度核查" {
          }
          frame "空白测试" {
          }
          frame "平行样测试" {
          }
          frame "加标回收" {
          }
          frame "空白校准" {
          }
          frame "标样校准" {
          }
        }
        n175 = Concatenate Strings(w175, "停止" ("字符串"), ">>" ("字符串")) -> (w173:string)
        n176 = Get Date/Time In Seconds() -> (seconds since 1Jan1904=w178:timestamp)
        n177 = Bundle By Name(cluster=T15 {"时间标识"=timestamp(0 s since 1904-01-01), "设备"="", "日志信息"="", "流程参数"=""} ("data in"), "时间标识"=w178, "设备"=w176, "日志信息"=w173) -> (w170:T15)
        n178 = call "总磷操作日志.vi"("data in"=w170) -> ()  [unwired: 11 in]
      }
    }
    n179 = case shown="真" w165 {
      tunnel: w134 -> [_ w383]
      frame False {
      }
      frame True {
        n180 = Subtract(x=w383, y=1) -> (x-y=w381:i32)
        n181 = Subtract(x=w381, y=5) -> (x-y=w385:i32)
        n182 = Greater Or Equal To 0?(x=w385) -> (x >= 0?=w384:bool)
        n183 = property on="多列列表框" class="MCListbox (严格)"() -> (error out=w389:errorcluster, "TopLeft"=w390:T17)  [unwired: 2 in, 1 out]
        n184 = Select(t=w385, s=w384, f=0) -> (s? t:f=w386:i32)
        n185 = Bundle By Name(cluster=w390, "Row"=w386) -> (w391:T17)
        n186 = property on="多列列表框" class="MCListbox (严格)"(error in=w389, "TopLeft"=w391) -> ()  [unwired: 1 in, 2 out]
      }
    }
    n187 = Or(x=w127, y=w164) -> (x .or. y?=w162:bool)
    n188 = Bundle By Name(cluster=T14 {"启动模式"=enum."跨度核查", "启动参数"=1, "量程"=enum."低量程"} ("参数簇"), "启动参数"=w158, "启动模式"=w160, "量程"=w159) -> (w152:T14)
    n189 = while {
      tunnel: w162 -> [w369]
      tunnel: w152 -> [w368]
      shift-right: [w363] -> _
      shift-left: _ -> [w365]
      shift-right: [w364] -> _
      shift-left: _ -> [w366]
      stop <- TRUE stop-if-true
      n190 = case shown="真" w369 {
        tunnel: [w371 w379] -> w364
        tunnel: [w370 w378] -> w363
        tunnel: w368 -> [_ w373]
        tunnel: w366 -> [w371 _]
        tunnel: w365 -> [w370 _]
        frame False {
        }
        frame True {
          n191 = call "斯坦道XML解析.vi"("添加的路径"="流程路径", "参数簇"=w373) -> ("步骤时间"=w374:string[], "步骤名"=w376:string[])  [unwired: 8 in]
          n192 = Build Array(w376, w374) -> (w375:string[][])
          n193 = for {
            tunnel: w376 -> [_] mode=indexing
            tunnel: [w380] -> w377 mode=indexing
            i -> [w380]
          }
          n194 = Transpose 2D Array(2D array=w375) -> (transposed array=w378:string[][])
          n195 = Number To Decimal String(number=w377) -> (decimal integer string=w379:string[])  [unwired: 1 in]
        }
      }
      n196 = property on="多列列表框" class="MCListbox (严格)"("ItemNames"=w363, "RowHdrs[]"=w364) -> ()  [unwired: 2 in, 2 out]
    }
    n197 = Wait (ms)(milliseconds to wait=u32 1000 ("等待时间（毫秒）")) -> ()  [unwired: 1 out]
  }
  n198 = while {
    stop <- FALSE stop-if-true
    n199 = Wait (ms)(milliseconds to wait=u32 1000 ("等待时间（毫秒）")) -> ()  [unwired: 1 out]
    n200 = global read "系统设置全局变量.vi" "三级权限"() -> (w395:bool)
    n201 = Select(t=T18."Enabled" ("禁用"), s=w395, f=T18."Disabled and Grayed Out" ("禁用")) -> (s? t:f=w392:T18)
    n202 = property on="设置" class="Bool"("DisabledEnum"=w392) -> ()  [unwired: 2 in, 2 out]
  }
  n203 = while {
    tunnel: w22 -> [w403]
    tunnel: w23 -> [_]
    stop <- FALSE stop-if-true
    n204 = Get Queue Status(queue=w403) -> (queue out=w399:refnum<queue>, # elements in queue=w398:i32)  [unwired: 2 in, 6 out]
    n205 = global read "总磷断电保存全局变量.vi" "流程路径"() -> (w402:path)
    n206 = global read "总磷断电保存全局变量.vi" "MB通信方式选择"() -> (w400:enum16{"串口", "TCP"})
    n207 = case shown="0" w398 {
      tunnel: w399 -> [_ w419]
      frame Default {
      }
      frame 0 {
        w417 = u16 1 items=["总磷"=1, "氨氮"=3] ("站号")
        # "试剂填充 172 \n管路清洗108\n氨氮92\n总磷131\n总磷海水147\n总氮76\n总氮海水92"
        n208 = global read "VAR总磷全局变量.vi" "状态告警区"() -> (w409:T6)
        n209 = Unbundle By Name(w409) -> ("系统时间"=w416:timestamp, "工作状态"=w408:T9)
        n210 = Bundle By Name(cluster=cluster{"命令":string, "data":variant} {"命令"="", "data"=variant} ("元素"), "命令"="读状态告警区", "data"=w417) -> (w421:cluster{"命令":string, "data":variant})
        n211 = Get Date/Time In Seconds() -> (seconds since 1Jan1904=w415:timestamp)
        n212 = Enqueue Element(queue=w419, element=w421) -> (queue out=w418:refnum<queue>)  [unwired: 2 in, 2 out]
        n213 = Subtract(x=w415, y=w416) -> (x-y=w414:dbl)
        n214 = Equal?(x=w408, y=T9."空闲") -> (x = y?=w406:bool)
        n215 = Absolute Value(x=w414) -> (abs(x)=w413:dbl)
        n216 = case shown="真" w406 {
          tunnel: w418 -> [w423 w426]
          tunnel: w417 -> [_ w425]
          tunnel: [w423 w424] -> w410
          frame False {
          }
          frame True {
            n217 = Bundle By Name(cluster=cluster{"命令":string, "data":variant} {"命令"="", "data"=variant} ("元素"), "命令"="读测量数据区", "data"=w425) -> (w428:cluster{"命令":string, "data":variant})
            n218 = Enqueue Element(queue=w426, element=w428) -> (queue out=w424:refnum<queue>)  [unwired: 2 in, 2 out]
          }
        }
        n219 = Greater Or Equal?(x=w413, y=120.0) -> (x >= y?=w411:bool)
        n220 = case shown="真" w411 {
          tunnel: w410 -> [_ w431]
          frame False {
          }
          frame True {
            n221 = call "总磷启动命令.vi"("参数"=T19 {"站号"=3, "量程切换"=enum."AUTO", "控制命令"=enum."校时", "模式设置"=enum."待机", "测量间隔"=0}) -> ("启动命令"=w430:cluster{"命令":string, "data":variant})  [unwired: 10 in]
            n222 = Enqueue Element(queue=w431, element=w430) -> ()  [unwired: 2 in, 3 out]
          }
        }
      }
    }
    n223 = local write "流程路径"(w402) -> ()
    n224 = case shown="\"TCP\"" w400 {
      tunnel: [w433 w434] -> w401
      frame "串口", Default {
        n225 = global read "总磷断电保存全局变量.vi" "VISA Resource"() -> (w433:refnum<visa-resource-name>)
      }
      frame "TCP" {
        n226 = global read "总磷断电保存全局变量.vi" "IP"() -> (w434:string)
      }
    }
    "字符串" <- w401
    n227 = Wait (ms)(milliseconds to wait=u32 1000 ("等待时间（毫秒）")) -> ()  [unwired: 1 out]
  }
  n228 = while {
    tunnel: w22 -> [w442]
    tunnel: w21 -> [w441]
    tunnel: w20 -> [w440]
    tunnel: w19 -> [w439]
    tunnel: w18 -> [w438]
    tunnel: w17 -> [w437]
    tunnel: w16 -> [w436]
    tunnel: w11 -> [_]
    tunnel: w7 -> [w435]
    stop <- FALSE stop-if-true
    n229 = event shown="[9] \"仪器参数设置\": 值改变" {
      selector: _ -> [_ _ _ _ _ _ _ _ _ _ _ _ _ _ _ _ _ _ _ _ _ _ _]
      dyn-events: _ -> [_ _ _ _ _ _ _ _ _ _ _ _ _ _ _ _ _ _ _ _ _ _ _]
      timeout: _ -> [_ _ _ _ _ _ _ _ _ _ _ _ _ _ _ _ _ _ _ _ _ _ _]
      tunnel: w442 -> [_ _ w458 w486 _ _ _ _ _ _ _ w594 w603 w610 _ _ _ _ _ _ _ _ _]
      tunnel: w441 -> [_ _ _ _ _ _ _ _ _ _ _ _ _ _ _ _ _ w626 _ w646 w655 w662 w674]
      tunnel: w440 -> [_ _ _ _ _ _ _ _ _ _ _ _ _ _ _ _ _ w624 _ w644 w657 w669 w680]
      tunnel: w439 -> [_ _ _ _ _ _ _ _ _ _ _ _ _ _ _ _ _ w625 _ w645 w656 w663 w675]
      tunnel: w438 -> [_ _ _ _ _ _ _ _ _ _ _ _ _ _ _ _ _ w620 _ _ _ _ _]
      tunnel: w437 -> [_ _ _ _ _ _ _ _ _ _ _ _ _ _ _ _ _ _ _ w640 _ _ _]
      tunnel: w436 -> [_ _ _ _ _ _ _ _ _ _ _ _ _ _ _ _ _ _ _ _ _ w667 _]
      tunnel: w435 -> [_ _ _ _ _ _ _ _ _ _ _ _ _ w605 _ _ _ _ _ _ _ _ _]
      tunnel: [_ w444 _ _ _ _ _ _ _ _ _ _ _ _ _ _ _ _ _ _ _ _ _] -> _
      event Timeout {
        n230 = event-data() -> ()  [unwired: 1 in, 3 out]
      }
      event "测量模式下拉列表", "量程下拉列表", "参数下拉列表": Value Change {
        n231 = event-data() -> ()  [unwired: 1 in, 6 out]
        n232 = local read "参数下拉列表"() -> (w446:enum16{"总磷", "总氮"})
        n233 = local read "测量模式下拉列表"() -> (w447:enum16{"水样测量", "零点核查", "跨度核查", "标样核查", "加标回收"})
        n234 = local read "量程下拉列表"() -> (w448:enum16{"低量程", "高量程"})
        n235 = Bundle("参数下拉列表"=w446, "测量模式下拉列表"=w447, "量程下拉列表"=w448) -> (w445:T13)  [unwired: 1 in]
        n236 = property on="曲线模型" class="曲线模型 (严格)"("属性"=w445) -> (error out=w444:errorcluster)  [unwired: 2 in, 1 out]
      }
      event "串口设置": Value Change {
        n237 = event-data() -> ()  [unwired: 1 in, 6 out]
        n238 = global read "总磷断电保存全局变量.vi" "VISA Resource"() -> (w455:refnum<visa-resource-name>)
        n239 = global read "总磷断电保存全局变量.vi" "MB通信方式选择"() -> (w449:enum16{"串口", "TCP"})
        n240 = global read "总磷断电保存全局变量.vi" "IP"() -> (w454:string)
        n241 = global read "总磷断电保存全局变量.vi" "PORT"() -> (w453:string)
        n242 = call "串口配置.vi"("PORT"=w453, "IP"=w454, "MB通信方式选择"=w449, "请选择串口:"=w455) -> ("PORT 2"=w451:string, "IP 2"=w452:string, "确认 2"=w456:bool, "VISA资源名称 2"=w457:refnum<visa-resource-name>, "MB通信方式选择 2"=w450:enum16{"串口", "TCP"})  [unwired: 3 in]
        n243 = case shown="真" w456 {
          tunnel: w457 -> [_ w463]
          tunnel: w458 -> [_ w462]
          tunnel: w452 -> [_ w461]
          tunnel: w451 -> [_ w460]
          tunnel: w450 -> [_ w459]
          frame False {
          }
          frame True {
            n244 = flat-sequence {
              tunnel: w463 -> [w468]
              tunnel: w462 -> [w469]
              tunnel: w461 -> [w467]
              tunnel: w460 -> [w466]
              tunnel: w459 -> [w465]
              frame #0 {
                n245 = global write "总磷断电保存全局变量.vi" "IP"(w467) -> ()
                n246 = global write "总磷断电保存全局变量.vi" "PORT"(w466) -> ()
                n247 = global write "总磷断电保存全局变量.vi" "MB通信方式选择"(w465) -> ()
                n248 = global write "总磷断电保存全局变量.vi" "VISA Resource"(w468) -> ()
                n249 = Flush Queue(queue=w469) -> (queue out=w464:refnum<queue>)  [unwired: 1 in, 2 out]
                n250 = Enqueue Element(queue=w464, element=cluster{"命令":string, "data":variant} {"命令"="启用模块", "data"=variant} ("元素")) -> ()  [unwired: 2 in, 3 out]
              }
              frame #1 {
                n251 = call <vilib>:"Application Directory.vi"() -> ("Application Directory"=w484:path)
                n252 = Build Path(base path=w484, name or relative path="data\\sys.ini" ("名称或相对路径")) -> (appended path=w482:path)
                n253 = call <vilib>:"Open Config Data.vi"("configuration file path"=w482) -> ("error out"=w478:errorcluster, "refnum"=w481:T7)  [unwired: 8 in, 1 out]
                n254 = vi-ref "总磷断电保存全局变量.vi"() -> (w480:refnum<vi>)
                n255 = call <userlib>:"Write Panel to INI__ogtk.vi"("error in (no error)"=w478, "VI ref"=w480, "refnum"=w481) -> ("error out"=w477:errorcluster, "refnum out"=w479:T7)  [unwired: 7 in]
                n256 = call <vilib>:"Close Config Data.vi"("error in (no error)"=w477, "refnum"=w479) -> ("error out"=w472:errorcluster, "file path"=w471:path)  [unwired: 8 in]
                n257 = Open/Create/Replace File(file path (use dialog)=w471, error in=w472) -> (refnum out=w475:refnum<file>, error out=w476:errorcluster)  [unwired: 4 in, 1 out]
                n258 = Flush File(refnum=w475, error in=w476) -> (refnum out=w474:refnum<file>, error out=w473:errorcluster)
                n259 = Close File(refnum=w474, error in=w473) -> ()  [unwired: 2 out]
              }
            }
          }
        }
      }
      event "模块启用": Value Change {
        n260 = event-data() -> ("OldVal"=w487:bool)  [unwired: 1 in, 5 out]
        n261 = Flush Queue(queue=w486) -> (queue out=w485:refnum<queue>)  [unwired: 1 in, 2 out]
        n262 = case shown="假" w487 {
          tunnel: w485 -> [w488 w490]
          frame False {
            n263 = Enqueue Element(queue=w488, element=cluster{"命令":string, "data":variant} {"命令"="停用模块", "data"=variant} ("元素")) -> ()  [unwired: 2 in, 3 out]
          }
          frame True {
            n264 = Enqueue Element(queue=w490, element=cluster{"命令":string, "data":variant} {"命令"="启用模块", "data"=variant} ("元素")) -> ()  [unwired: 2 in, 3 out]
          }
        }
      }
      event "流程路径": Value Change {
        n265 = event-data() -> ()  [unwired: 1 in, 6 out]
        n266 = flat-sequence {
          frame #0 {
            n267 = local read "流程路径"() -> (w492:path)
            n268 = global write "总磷断电保存全局变量.vi" "流程路径"(w492) -> ()
          }
          frame #1 {
            n269 = call <vilib>:"Application Directory.vi"() -> ("Application Directory"=w506:path)
            n270 = Build Path(base path=w506, name or relative path="data\\sys.ini" ("名称或相对路径")) -> (appended path=w504:path)
            n271 = call <vilib>:"Open Config Data.vi"("configuration file path"=w504) -> ("error out"=w500:errorcluster, "refnum"=w503:T7)  [unwired: 8 in, 1 out]
            n272 = vi-ref "总磷断电保存全局变量.vi"() -> (w502:refnum<vi>)
            n273 = call <userlib>:"Write Panel to INI__ogtk.vi"("error in (no error)"=w500, "VI ref"=w502, "refnum"=w503) -> ("error out"=w499:errorcluster, "refnum out"=w501:T7)  [unwired: 7 in]
            n274 = call <vilib>:"Close Config Data.vi"("error in (no error)"=w499, "refnum"=w501) -> ("error out"=w494:errorcluster, "file path"=w493:path)  [unwired: 8 in]
            n275 = Open/Create/Replace File(file path (use dialog)=w493, error in=w494) -> (refnum out=w497:refnum<file>, error out=w498:errorcluster)  [unwired: 4 in, 1 out]
            n276 = Flush File(refnum=w497, error in=w498) -> (refnum out=w496:refnum<file>, error out=w495:errorcluster)
            n277 = Close File(refnum=w496, error in=w495) -> ()  [unwired: 2 out]
          }
        }
      }
      event "公式一键写入": Value Change {
        n278 = event-data() -> ()  [unwired: 1 in, 6 out]
        n279 = local read "公式"() -> (w507:cluster{"X^2":dbl, "X":dbl, "b":dbl})
        n280 = call "公式复合写入.vi"("公式"=w507) -> ()  [unwired: 11 in]
      }
      event "备用系数一键写入": Value Change {
        n281 = event-data() -> ()  [unwired: 1 in, 6 out]
        n282 = local read "备用系数"() -> (w508:T4)
        n283 = call "量程参数复合参数写入.vi"("备用系数"=w508) -> ()  [unwired: 11 in]
      }
      event "曲线模型": Value Change {
        n284 = event-data() -> ()  [unwired: 1 in, 6 out]
        n285 = Unbundle By Name("曲线模型") -> ("X^2"=w511:dbl, "X"=w510:dbl, "B"=w509:dbl)
        n286 = local read "公式"() -> (w514:cluster{"X^2":dbl, "X":dbl, "b":dbl})
        n287 = Bundle By Name(cluster=w514, "X^2"=w511, "X"=w510, "b"=w509) -> (w513:cluster{"X^2":dbl, "X":dbl, "b":dbl})
        n288 = local write "公式"(w513) -> ()
      }
      event "质控参数设置": Value Change {
        n289 = event-data() -> ()  [unwired: 1 in, 6 out]
        n290 = global read "总磷断电保存全局变量.vi" "质控参数设置"() -> (w515:T20)
        n291 = call "总磷质控参数设置.vi"("质控参数设置"=w515) -> ("输出簇"=w516:T21)  [unwired: 10 in]
        n292 = Unbundle By Name(w516) -> ("确定"=w517:bool)
        n293 = case shown="真" w517 {
          tunnel: w516 -> [_ w519]
          tunnel: w515 -> [_ w518]
          frame False {
          }
          frame True {
            n294 = flat-sequence {
              tunnel: w519 -> [w526]
              tunnel: w518 -> [w525]
              frame #0 {
                n295 = Unbundle By Name(w526) -> ("总磷跨度值"=w524:dbl, "总磷零点标准液浓度"=w523:dbl, "总磷跨度标准液浓度"=w522:dbl, "总磷标准液标准浓度"=w521:dbl)
                n296 = Bundle By Name(cluster=w525, "总磷跨度值"=w524, "总磷零点标准液浓度"=w523, "总磷跨度标准液浓度"=w522, "总磷标准液标准浓度"=w521) -> (w520:T20)
                n297 = global write "总磷断电保存全局变量.vi" "质控参数设置"(w520) -> ()
              }
              frame #1 {
                n298 = call <vilib>:"Application Directory.vi"() -> ("Application Directory"=w540:path)
                n299 = Build Path(base path=w540, name or relative path="data\\sys.ini" ("名称或相对路径")) -> (appended path=w538:path)
                n300 = call <vilib>:"Open Config Data.vi"("configuration file path"=w538) -> ("error out"=w534:errorcluster, "refnum"=w537:T7)  [unwired: 8 in, 1 out]
                n301 = vi-ref "总磷断电保存全局变量.vi"() -> (w536:refnum<vi>)
                n302 = call <userlib>:"Write Panel to INI__ogtk.vi"("error in (no error)"=w534, "VI ref"=w536, "refnum"=w537) -> ("error out"=w533:errorcluster, "refnum out"=w535:T7)  [unwired: 7 in]
                n303 = call <vilib>:"Close Config Data.vi"("error in (no error)"=w533, "refnum"=w535) -> ("error out"=w528:errorcluster, "file path"=w527:path)  [unwired: 8 in]
                n304 = Open/Create/Replace File(file path (use dialog)=w527, error in=w528) -> (refnum out=w531:refnum<file>, error out=w532:errorcluster)  [unwired: 4 in, 1 out]
                n305 = Flush File(refnum=w531, error in=w532) -> (refnum out=w530:refnum<file>, error out=w529:errorcluster)
                n306 = Close File(refnum=w530, error in=w529) -> ()  [unwired: 2 out]
              }
            }
          }
        }
      }
      event "仪器参数设置": Value Change {
        n307 = event-data() -> ()  [unwired: 1 in, 6 out]
        n308 = global read "总磷断电保存全局变量.vi" "总磷仪器参数"() -> (w542:T22)
        n309 = call "仪器参数设置.vi"("总磷仪器参数"=w542) -> ("总磷仪器参数输出"=w541:T23)  [unwired: 10 in]
        n310 = Unbundle By Name(w541) -> ("确定"=w543:bool)
        n311 = case shown="真" w543 {
          tunnel: w541 -> [_ w545]
          tunnel: w542 -> [_ w544]
          frame False {
          }
          frame True {
            n312 = flat-sequence {
              tunnel: w545 -> [w562]
              tunnel: w544 -> [w561]
              frame #0 {
                n313 = Unbundle By Name(w562) -> ("测量量程"=w560:dbl, "测量精度"=w559:dbl, "测量间隔"=w558:dbl, "消解温度"=w557:dbl, "消解时长"=w555:dbl, "空白校准时间"=w554:timestamp, "曲线截距"=w553:dbl, "曲线斜率"=w552:dbl, "测量检出限"=w551:dbl, "测量信号值"=w550:dbl, "线性相关系数"=w549:dbl, "二次多项式系数"=w548:dbl, "标样校准时间"=w547:timestamp, "稀释倍数"=w546:dbl)
                n314 = Bundle By Name(cluster=w561, "测量量程"=w560, "测量精度"=w559, "测量间隔"=w558, "消解温度"=w557, "消解时长"=w555, "空白校准时间"=w554, "曲线截距"=w553, "曲线斜率"=w552, "测量检出限"=w551, "测量信号值"=w550, "线性相关系数"=w549, "二次多项式系数"=w548, "标样校准时间"=w547, "稀释倍数"=w546) -> (w556:T22)
                n315 = global write "总磷断电保存全局变量.vi" "总磷仪器参数"(w556) -> ()
              }
              frame #1 {
                n316 = call <vilib>:"Application Directory.vi"() -> ("Application Directory"=w576:path)
                n317 = Build Path(base path=w576, name or relative path="data\\sys.ini" ("名称或相对路径")) -> (appended path=w574:path)
                n318 = call <vilib>:"Open Config Data.vi"("configuration file path"=w574) -> ("error out"=w570:errorcluster, "refnum"=w573:T7)  [unwired: 8 in, 1 out]
                n319 = vi-ref "总磷断电保存全局变量.vi"() -> (w572:refnum<vi>)
                n320 = call <userlib>:"Write Panel to INI__ogtk.vi"("error in (no error)"=w570, "VI ref"=w572, "refnum"=w573) -> ("error out"=w569:errorcluster, "refnum out"=w571:T7)  [unwired: 7 in]
                n321 = call <vilib>:"Close Config Data.vi"("error in (no error)"=w569, "refnum"=w571) -> ("error out"=w564:errorcluster, "file path"=w563:path)  [unwired: 8 in]
                n322 = Open/Create/Replace File(file path (use dialog)=w563, error in=w564) -> (refnum out=w567:refnum<file>, error out=w568:errorcluster)  [unwired: 4 in, 1 out]
                n323 = Flush File(refnum=w567, error in=w568) -> (refnum out=w566:refnum<file>, error out=w565:errorcluster)
                n324 = Close File(refnum=w566, error in=w565) -> ()  [unwired: 2 out]
              }
            }
          }
        }
      }
      event "总磷自动测试量程配置": Value Change {
        n325 = event-data() -> ()  [unwired: 1 in, 6 out]
        n326 = flat-sequence {
          frame #0 {
            n327 = global write "总磷断电保存全局变量.vi" "总磷自动测试量程配置"("总磷自动测试量程配置") -> ()
          }
          frame #1 {
            n328 = call <vilib>:"Application Directory.vi"() -> ("Application Directory"=w591:path)
            n329 = Build Path(base path=w591, name or relative path="data\\sys.ini" ("名称或相对路径")) -> (appended path=w589:path)
            n330 = call <vilib>:"Open Config Data.vi"("configuration file path"=w589) -> ("error out"=w585:errorcluster, "refnum"=w588:T7)  [unwired: 8 in, 1 out]
            n331 = vi-ref "总磷断电保存全局变量.vi"() -> (w587:refnum<vi>)
            n332 = call <userlib>:"Write Panel to INI__ogtk.vi"("error in (no error)"=w585, "VI ref"=w587, "refnum"=w588) -> ("error out"=w584:errorcluster, "refnum out"=w586:T7)  [unwired: 7 in]
            n333 = call <vilib>:"Close Config Data.vi"("error in (no error)"=w584, "refnum"=w586) -> ("error out"=w579:errorcluster, "file path"=w578:path)  [unwired: 8 in]
            n334 = Open/Create/Replace File(file path (use dialog)=w578, error in=w579) -> (refnum out=w582:refnum<file>, error out=w583:errorcluster)  [unwired: 4 in, 1 out]
            n335 = Flush File(refnum=w582, error in=w583) -> (refnum out=w581:refnum<file>, error out=w580:errorcluster)
            n336 = Close File(refnum=w581, error in=w580) -> ()  [unwired: 2 out]
          }
        }
      }
      event "手动启动": Value Change {
        n337 = event-data() -> ()  [unwired: 1 in, 6 out]
        n338 = call "总磷启动参数对话框.vi"() -> ("确认"=w592:bool, "元素"=w593:cluster{"命令":string, "data":variant})  [unwired: 10 in]
        n339 = case shown="真" w592 {
          tunnel: w594 -> [_ w596]
          tunnel: w593 -> [_ w595]
          frame False {
          }
          frame True {
            n340 = Enqueue Element(queue=w596, element=w595) -> ()  [unwired: 2 in, 3 out]
          }
        }
      }
      event "单步测试": Value Change {
        w598 = u16 1 items=["总磷"=1, "氨氮"=3] ("站号")
        n341 = event-data() -> ()  [unwired: 1 in, 6 out]
        n342 = Bundle("站号"=w598, "总磷氨氮调试"="总磷氨氮调试") -> (w597:cluster{"站号":u16, "总磷氨氮调试":u16[]})  [unwired: 1 in]
        n343 = Bundle By Name(cluster=cluster{"命令":string, "data":variant} {"命令"="", "data"=variant} ("元素"), "命令"="debug", "data"=w597) -> (w600:cluster{"命令":string, "data":variant})
        n344 = Enqueue Element(queue=w603, element=w600) -> ()  [unwired: 2 in, 3 out]
      }
      event "停止": Value Change {
        n345 = event-data() -> ()  [unwired: 1 in, 6 out]
        n346 = Cancel Notification(0:w605) -> (8:w606:refnum<notifier>)  [unwired: 1 in, 2 out]
        n347 = Enqueue Element(queue=w610, element=cluster{"命令":string, "data":variant} {"命令"="启动", "data"=variant(cluster{"站号":u16, "控制命令输出":u16[]} {"站号"=1, "控制命令输出"=[2816]})} ("元素")) -> (queue out=w607:refnum<queue>)  [unwired: 2 in, 2 out]
        n348 = Send Notification(notification=TRUE ("通知"), notifier=w606) -> ()  [unwired: 1 in, 2 out]
        n349 = Enqueue Element(queue=w607, element=cluster{"命令":string, "data":variant} {"命令"="启动", "data"=variant(cluster{"站号":u16, "控制命令输出":u16[]} {"站号"=2, "控制命令输出"=[2816]})} ("元素")) -> ()  [unwired: 2 in, 3 out]
      }
      event "设置": Value Change {
        n350 = event-data() -> ()  [unwired: 1 in, 6 out]
        n351 = property on="窗格" class="Pane"("Origin"=T8 {"Horizontal"=0, "Vertical"=628} ("原点")) -> ()  [unwired: 2 in, 2 out]
      }
      event "返回": Value Change {
        n352 = event-data() -> ()  [unwired: 1 in, 6 out]
        n353 = property on="窗格" class="Pane"("Origin"=T8 {"Horizontal"=0, "Vertical"=0} ("原点")) -> ()  [unwired: 2 in, 2 out]
      }
      event "公式.X^2", "公式.X", "公式.b", "量程切换阈值.阈值", "量程切换阈值.标液浓度", "备用系数.量程上限", "备用系数.量程下限", "备用系数.检出限", "备用系数.精度": Mouse Down {
        n354 = event-data() -> ("CtlRef"=w616:refnum<vi>)  [unwired: 1 in, 5 out]
        n355 = property class="DigNum (严格)"(reference=w616) -> (reference out=w614:refnum<vi>, "Value"=w615:dbl)  [unwired: 1 in, 1 out]
        n356 = call "数字键盘.vi"("OldNumber"=w615) -> ("NewNumber"=w613:dbl)
        n357 = property class="DigNum (严格)"(reference=w614, "Val(Sgnl)"=w613) -> ()  [unwired: 1 in, 2 out]
      }
      event "读公式": Value Change {
        n358 = event-data() -> ()  [unwired: 1 in, 6 out]
        n359 = property class="Enum (严格)"(reference=w624) -> ("Value"=w623:enum16{"总磷", "总氮"})  [unwired: 1 in, 2 out]
        n360 = property class="Enum (严格)"(reference=w625) -> ("Value"=w622:enum16{"水样测量", "零点核查", "跨度核查", "标样核查", "加标回收"})  [unwired: 1 in, 2 out]
        n361 = property class="Enum (严格)"(reference=w626) -> ("Value"=w621:enum16{"低量程", "高量程"})  [unwired: 1 in, 2 out]
        n362 = call "总磷总氮公式读取.vi"("量程"=w621, "测量模式"=w622, "测量参数"=w623) -> ("error out"=w618:errorcluster, "公式"=w619:cluster{"X^2":dbl, "X":dbl, "b":dbl})  [unwired: 7 in]
        n363 = property class="Clust (严格)"(reference=w620, "Value"=w619) -> ()  [unwired: 1 in, 2 out]
        n364 = case shown="错误" w618 {
          tunnel: ["读取成功" ("消息") "读取失败" ("消息")] -> w617
          frame No Error {
          }
          frame Error {
          }
        }
        n365 = One Button Dialog(message=w617) -> ()  [unwired: 1 in, 1 out]
      }
      event "写公式": Value Change {
        n366 = event-data() -> ()  [unwired: 1 in, 6 out]
        n367 = call "总磷总氮公式写入.vi"("公式"="公式", "量程"="量程下拉列表", "测量模式"="测量模式下拉列表", "测量参数"="参数下拉列表") -> ("error out"=w631:errorcluster)  [unwired: 7 in]
        n368 = case shown="无错误" w631 {
          tunnel: ["写入成功" ("消息") "写入失败" ("消息")] -> w632
          frame No Error {
          }
          frame Error {
          }
        }
        n369 = One Button Dialog(message=w632) -> ()  [unwired: 1 in, 1 out]
      }
      event "量程切换阈值读取": Value Change {
        n370 = event-data() -> ()  [unwired: 1 in, 6 out]
        n371 = property class="Enum (严格)"(reference=w644) -> ("Value"=w643:enum16{"总磷", "总氮"})  [unwired: 1 in, 2 out]
        n372 = property class="Enum (严格)"(reference=w645) -> ("Value"=w642:enum16{"水样测量", "零点核查", "跨度核查", "标样核查", "加标回收"})  [unwired: 1 in, 2 out]
        n373 = property class="Enum (严格)"(reference=w646) -> ("Value"=w641:enum16{"低量程", "高量程"})  [unwired: 1 in, 2 out]
        n374 = call "总磷总氮量程读取.vi"("量程"=w641, "测量模式"=w642, "测量参数"=w643) -> ("error out"=w637:errorcluster, "量程切换阈值"=w639:cluster{"阈值":dbl, "标液浓度":dbl})  [unwired: 7 in]
        n375 = property class="Clust (严格)"(reference=w640, "Value"=w639) -> ()  [unwired: 1 in, 2 out]
        n376 = case shown="错误" w637 {
          tunnel: ["读取成功" ("消息") "读取失败" ("消息")] -> w638
          frame No Error {
          }
          frame Error {
          }
        }
        n377 = One Button Dialog(message=w638) -> ()  [unwired: 1 in, 1 out]
      }
      event "量程切换阈值写入": Value Change {
        n378 = event-data() -> ()  [unwired: 1 in, 6 out]
        n379 = property class="Enum (严格)"(reference=w657) -> ("Value"=w654:enum16{"总磷", "总氮"})  [unwired: 1 in, 2 out]
        n380 = property class="Enum (严格)"(reference=w656) -> ("Value"=w653:enum16{"水样测量", "零点核查", "跨度核查", "标样核查", "加标回收"})  [unwired: 1 in, 2 out]
        n381 = property class="Enum (严格)"(reference=w655) -> ("Value"=w652:enum16{"低量程", "高量程"})  [unwired: 1 in, 2 out]
        n382 = call "总磷总氮量程写入.vi"("量程切换阈值"="量程切换阈值", "量程"=w652, "测量模式"=w653, "测量参数"=w654) -> ("error out"=w649:errorcluster)  [unwired: 7 in]
        n383 = case shown="无错误" w649 {
          tunnel: ["写入成功" ("消息") "写入失败" ("消息")] -> w650
          frame No Error {
          }
          frame Error {
          }
        }
        n384 = One Button Dialog(message=w650) -> ()  [unwired: 1 in, 1 out]
      }
      event "备用系数读取": Value Change {
        n385 = event-data() -> ()  [unwired: 1 in, 6 out]
        n386 = property class="Enum (严格)"(reference=w669) -> ("Value"=w668:enum16{"总磷", "总氮"})  [unwired: 1 in, 2 out]
        n387 = property class="Enum (严格)"(reference=w663) -> ("Value"=w661:enum16{"水样测量", "零点核查", "跨度核查", "标样核查", "加标回收"})  [unwired: 1 in, 2 out]
        n388 = property class="Enum (严格)"(reference=w662) -> ("Value"=w660:enum16{"低量程", "高量程"})  [unwired: 1 in, 2 out]
        n389 = call "总磷总氮备用系数读取.vi"("量程"=w660, "测量模式"=w661, "测量参数"=w668) -> ("error out"=w664:errorcluster, "备用系数"=w666:T4)  [unwired: 7 in]
        n390 = property class="Clust (严格)"(reference=w667, "Value"=w666) -> ()  [unwired: 1 in, 2 out]
        n391 = case shown="错误" w664 {
          tunnel: ["读取成功" ("消息") "读取失败" ("消息")] -> w665
          frame No Error {
          }
          frame Error {
          }
        }
        n392 = One Button Dialog(message=w665) -> ()  [unwired: 1 in, 1 out]
      }
      event "备用系数写入": Value Change {
        n393 = event-data() -> ()  [unwired: 1 in, 6 out]
        n394 = property class="Enum (严格)"(reference=w680) -> ("Value"=w679:enum16{"总磷", "总氮"})  [unwired: 1 in, 2 out]
        n395 = property class="Enum (严格)"(reference=w675) -> ("Value"=w673:enum16{"水样测量", "零点核查", "跨度核查", "标样核查", "加标回收"})  [unwired: 1 in, 2 out]
        n396 = property class="Enum (严格)"(reference=w674) -> ("Value"=w672:enum16{"低量程", "高量程"})  [unwired: 1 in, 2 out]
        n397 = call "总磷总氮备用系数写入.vi"("备用系数"="备用系数", "量程"=w672, "测量模式"=w673, "测量参数"=w679) -> ("error out"=w676:errorcluster)  [unwired: 7 in]
        n398 = case shown="无错误" w676 {
          tunnel: ["写入成功" ("消息") "写入失败" ("消息")] -> w677
          frame No Error {
          }
          frame Error {
          }
        }
        n399 = One Button Dialog(message=w677) -> ()  [unwired: 1 in, 1 out]
      }
    }
  }
